vi "Pick&Place_ladder_shih_v5_peek.vi"() -> ()   [LabVIEW 2016]
uses:
  Classes/Controllers/I-O/Copy of NI-DAQ Folder/NI-DAQ.lvclass
  D:/INTT/V1/Classes/Controllers/I-O/Copy of I-O Folder/I-O.lvclass
  Classes/Controllers/Dispenser/Copy of Ultimus V2 Folder/Ultimus V2.lvclass
  <vilib>/Analysis/coordinate.llb/2D Cartesian Coordinate Rotation (Scalar).vi
  <vilib>/Utility/file.llb/Read Delimited Spreadsheet (DBL).vi
  <vilib>/Utility/file.llb/Write Delimited Spreadsheet (DBL).vi
  Classes/Controllers/Motion/Copy of Motion Folder/Motion.lvclass
  Classes/Controllers/Camera/Copy of Controller Folder/Controller.lvclass
  <vilib>/Analysis/NI_AALPro.lvlib
  Classes/Controllers/I-O/Copy of I-O Folder/I-O.lvclass
panel:
  out "chip distance":dbl format="%#_8g"
  out "after SL":dbl[](array[numeric]) format="%#_8g"
  in  "module placing offset":dbl[][](array[numeric])=[[0.0, -0.1, 0.0, 0.0], [0.0, -0.1, 0.0, 0.0]]
  out "after SR":dbl[](array[numeric]) format="%#_8g"
  out "after NL":dbl[](array[numeric]) format="%#_8g"
  out "S chip":dbl[](array[numeric]) format="%#_8g"
  out "N chip":dbl[](array[numeric]) format="%#_8g"
  in  "file path (dialog if empty) 2":path=path "C:/Users/PAGANIS/Desktop/shih cheng wei/OGP/test1-2.txt"
  out "bless from OGP !!! Center of  stave":dbl[](array[numeric])
  out "bless from OGP !! measured stave size":dbl[](array[numeric])
  in  "Bless from OGP":bool
  out "FROM Detail !!! Center of module on stave":dbl[](array[numeric])
  out "FROM Detail !! measured stave size":dbl[](array[numeric])
  in  "Align Stave in detail":bool
  in  "check height?":bool
  in  "Uttimus presssure":i64=10
  out "Status":bool
  out "measured HDI top-left position":dbl[][](array[numeric])
  in  "HDI vacuum channel":i32=18
  in  "vacuum":bool=TRUE
  in  "HDI vacuum":bool
  out "measured stave size":dbl[](array[numeric])
  out "Stave mark":dbl[][](array[numeric])
  out "Center of module on stave":dbl[](array[numeric])
  out "Center of HDI from alignment mark":dbl[](array[numeric])
  out "Measured HDI size":dbl[][](array[numeric])
  out "module position on stave":dbl[][](array[numeric])
  in  "Default Stave dimension":dbl[](array[numeric])=[34.0, 472.0, -0.335295, -0.000320234]
  in  "Default Stave upper left mark":dbl[](array[numeric])=[584.376, 675.576, 70.9882, 0.000840064]
  out "Needle parking position":dbl[](array[numeric])
  in  "Uppler / Lower Stave":bool=TRUE
  out "Gantry current position":dbl[](array[numeric])
  in  "READ Position":bool
  in  "Needle Height Compenstation\n(glue gap)":dbl=0.33
  in  "Needle Alignment":bool
  in  "Parking position":dbl[](array[numeric])=[625.0, 625.0, 0.0, 0.01]
  in  "GOTO":bool
  in  "Default Pickup Tool Position":dbl[][](array[numeric])=[[152.226, 682.729, 36.8129, -0.0151898], [700.0, 800.0, 20.0, 0.01]]
  in  "Number of module \nto be assembled":i32=1
  in  "Default HDI alignment \nmark position":dbl[](array[numeric])=[448.322, 976.582, 74.9872, 0.000191129]
  in  "Default HDI size":dbl[](array[numeric])=[24.2437, 231.446, -0.099339, 0.000191129]
  out "# of tasks excuted":i32
  out "module on tray position":dbl[][](array[numeric])
  out "PickupTool \nCenterPosition":dbl[](array[numeric])
  in  "Inititalize":bool
  in  "Pick and place":bool
  in  "Deposit Glue":bool
  in  "Measure Pickup Tools":bool
  in  "Align Stave":bool
  out "default module position on stave":dbl[][](array[numeric])
  in  "Stop":bool
  in  "Measure HDI":bool
  # "Ladder Assembly"
  # "Lower\nmodule"
  # "Upper\nmodule"
  # "Sensor 0.32 -> 200 micron glue thickness\nChips 0.37-> 140 micron glue thickness"
  # "ACTIONS"
  # "Stave infomation"
  # "Module infomation"
  # "Pick and Place"
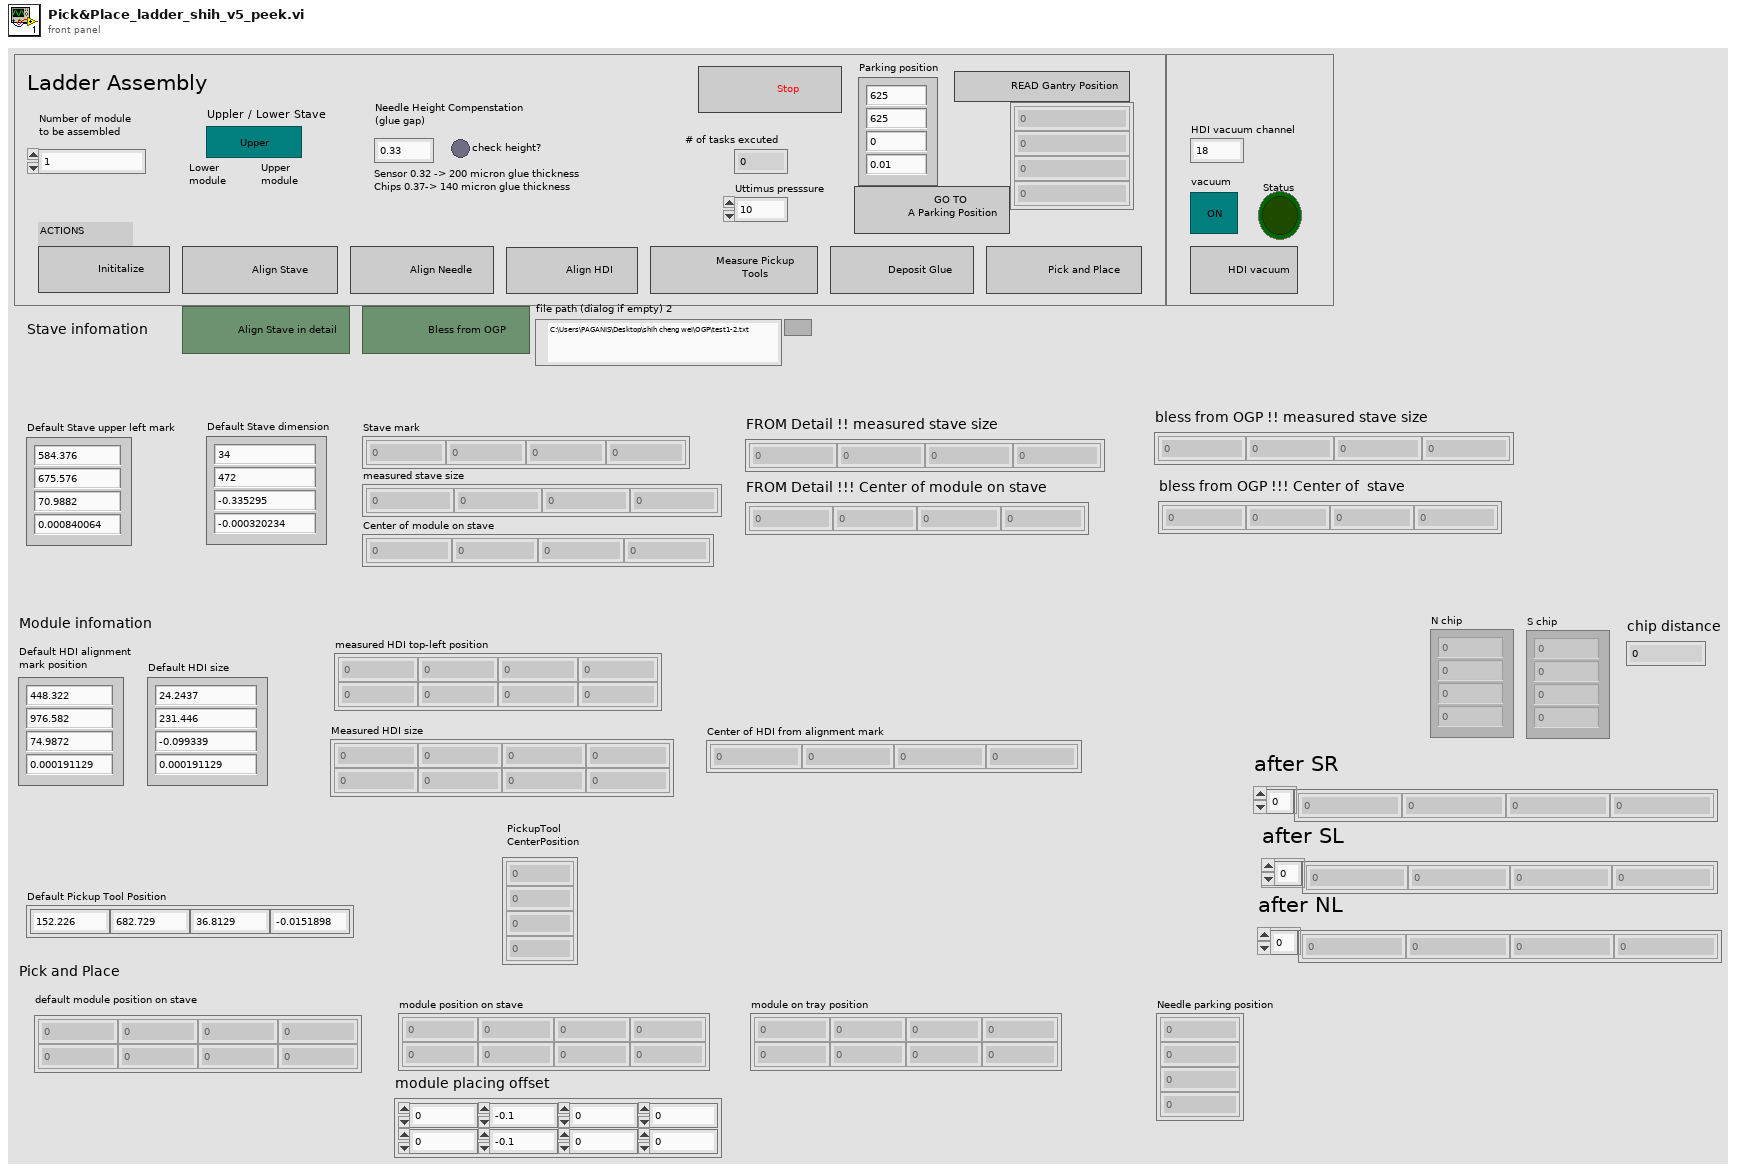
[diagram p1: front panel]
types:
  T1 = typedef "Controller.lvclass/Controllers.ctl" = cluster{"Copy of Motion.lvclass":refnum<class "Motion.lvclass">, "Copy of I-O.lvclass":refnum<class "I-O.lvclass">, "Copy of Dispenser.lvclass":refnum<class "Dispenser.lvclass">}
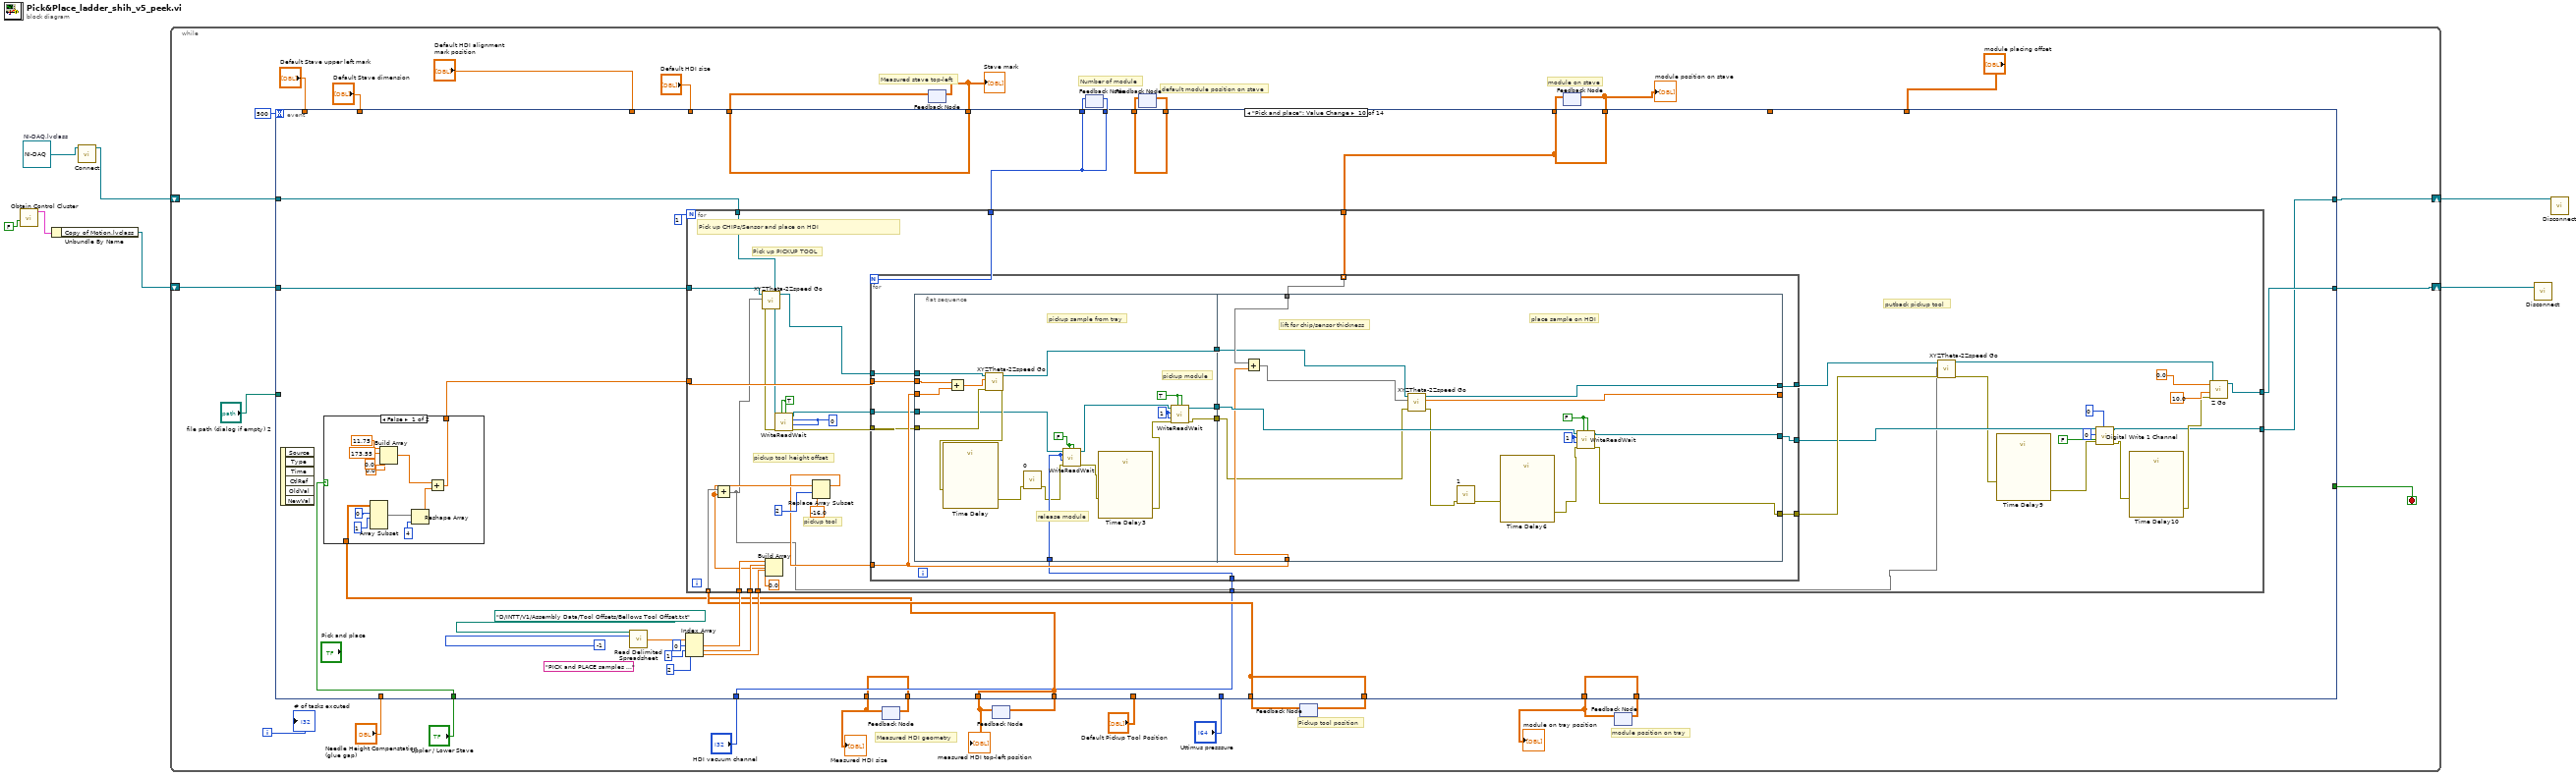
[diagram p0: block diagram]
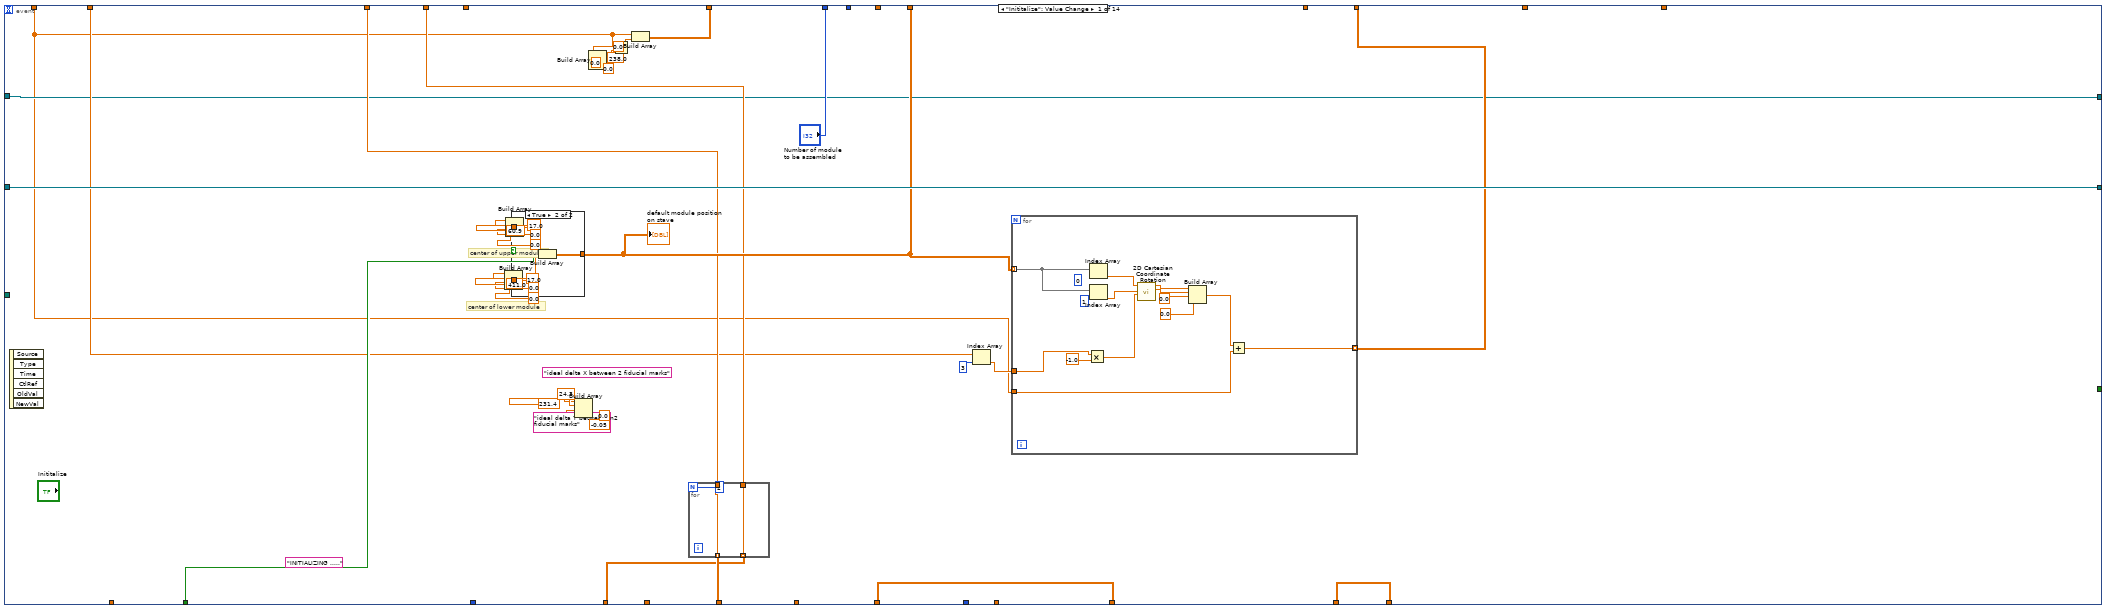
[diagram p2: hidden frame]
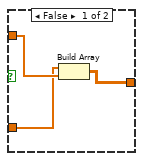
[diagram p3: hidden frame]
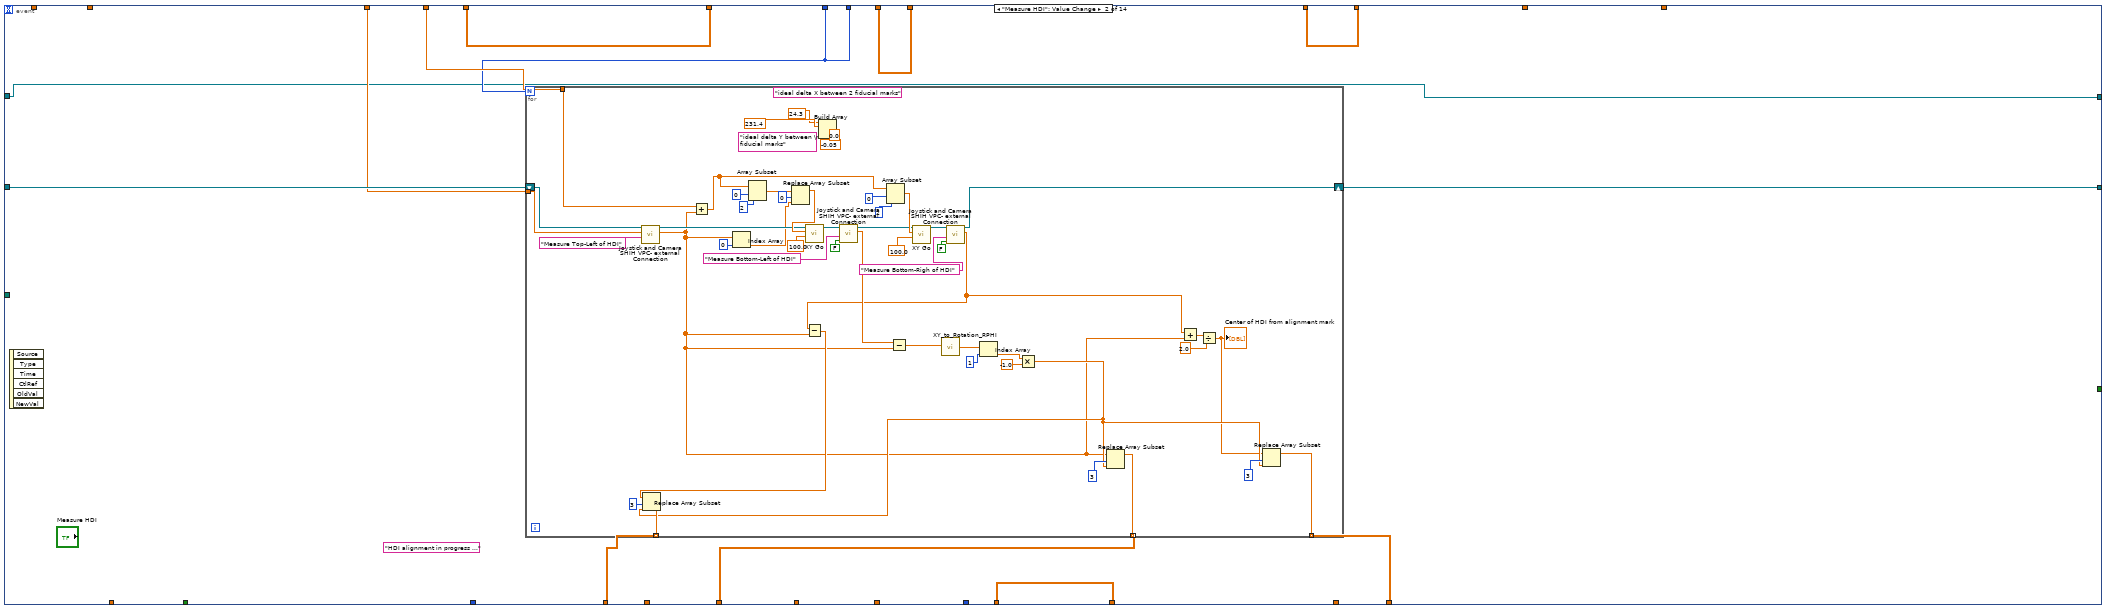
[diagram p4: hidden frame]
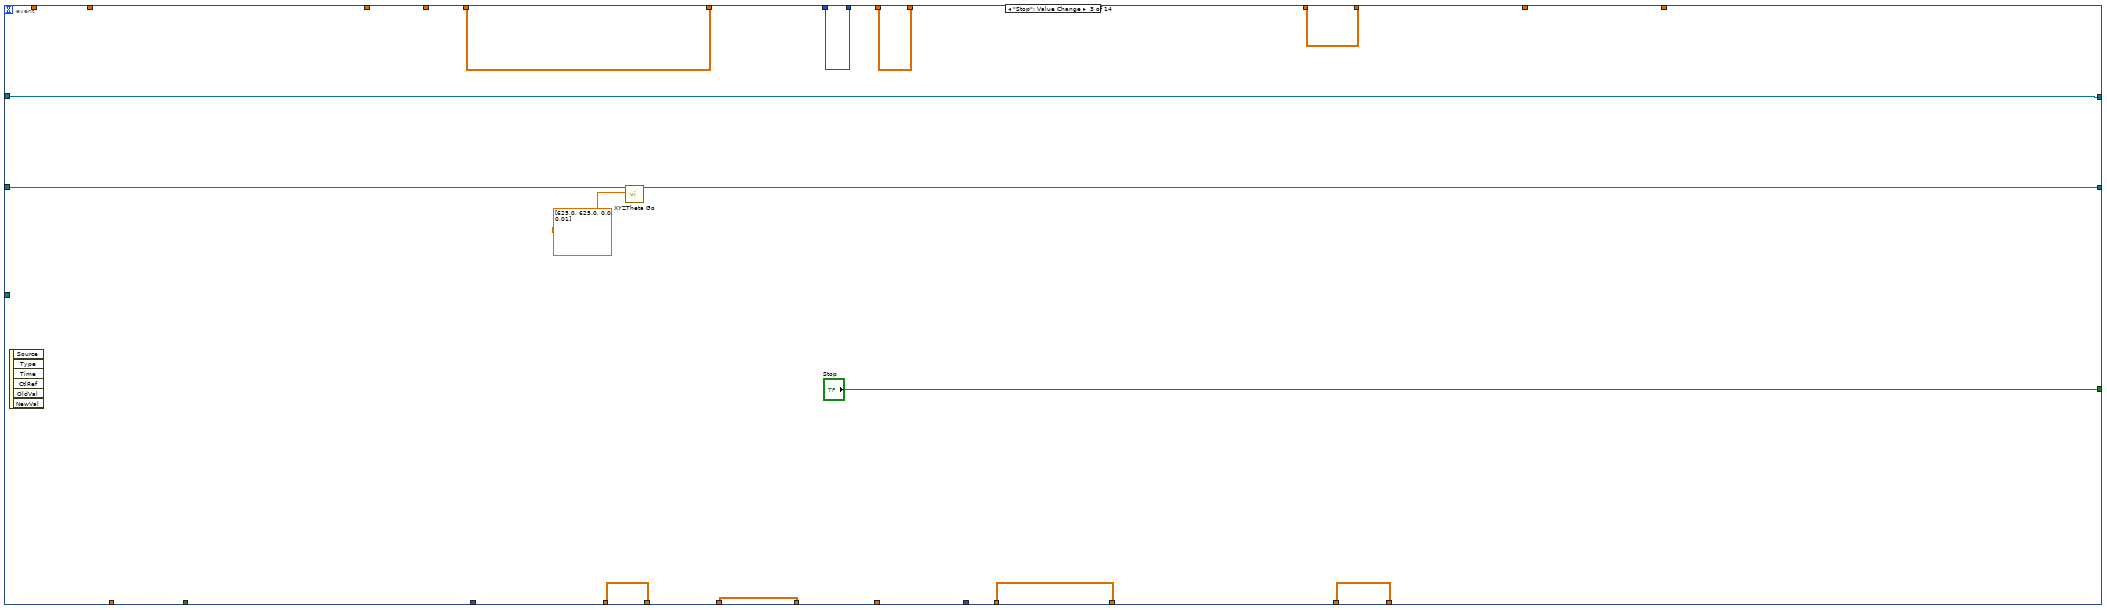
[diagram p5: hidden frame]
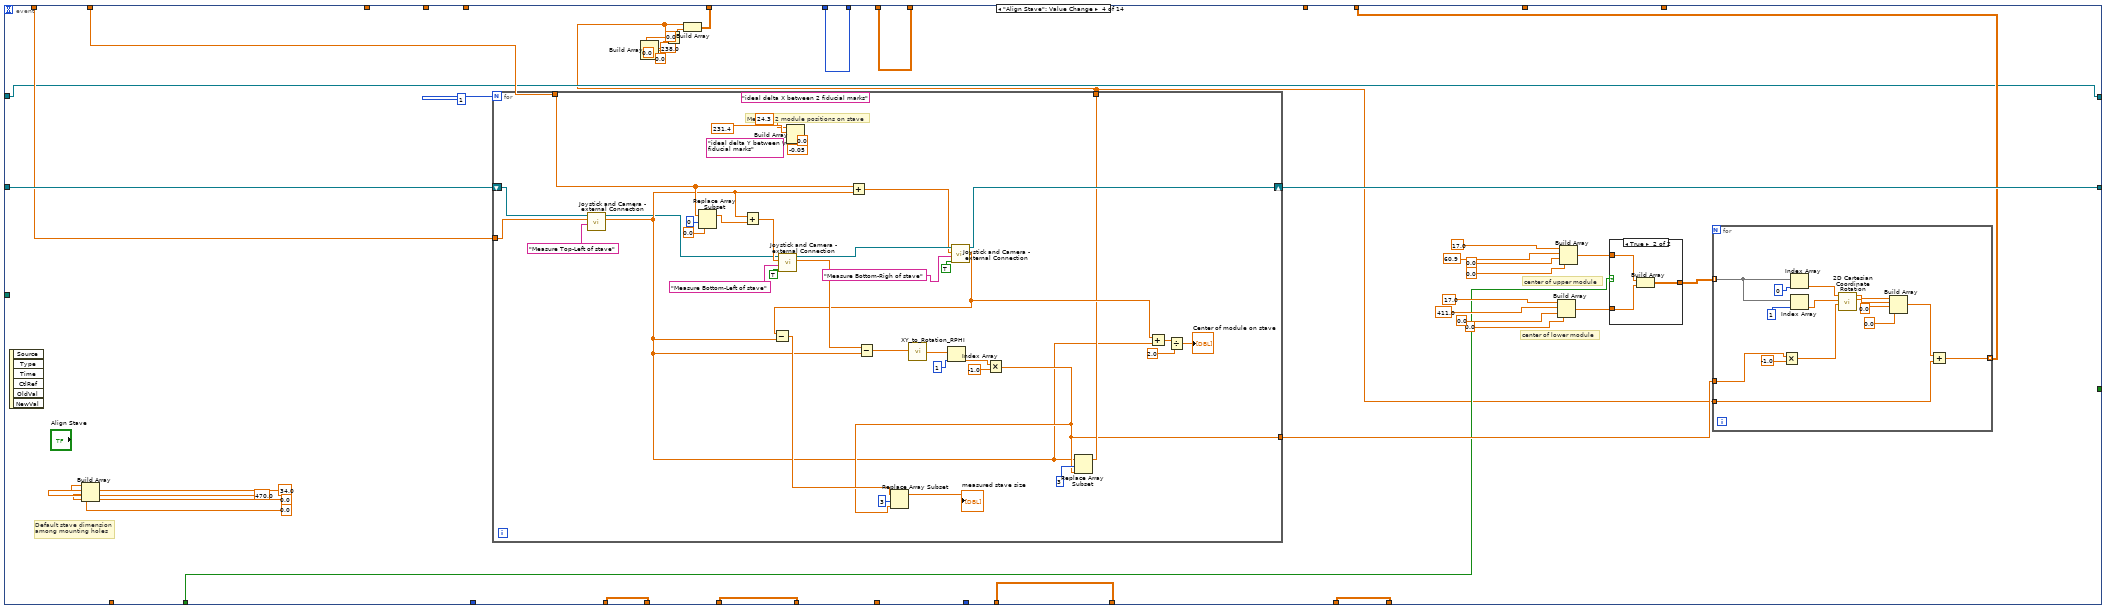
[diagram p6: hidden frame]
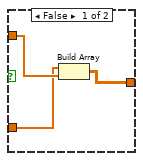
[diagram p7: hidden frame]
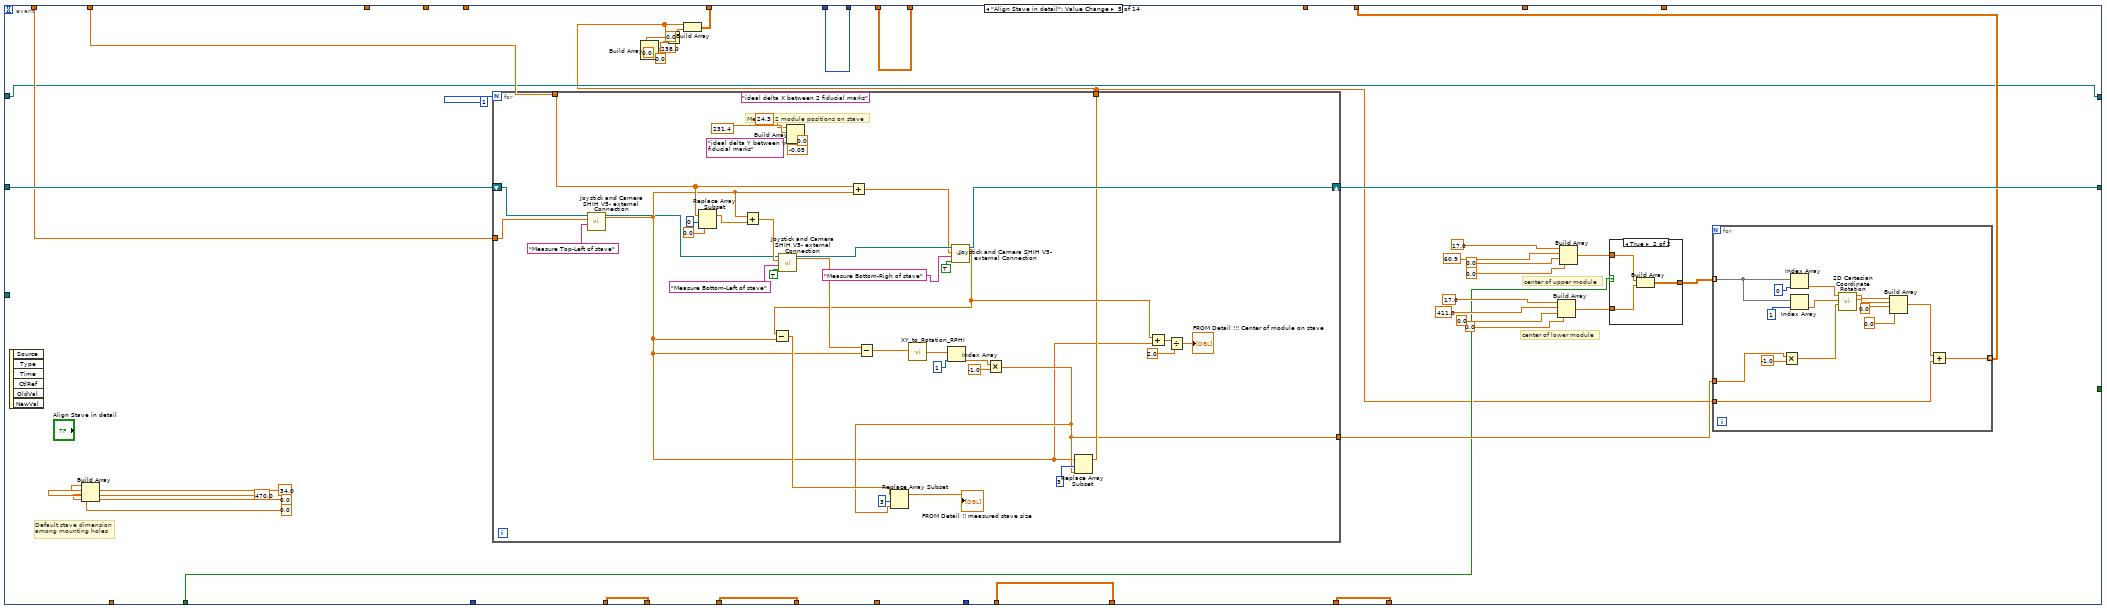
[diagram p8: hidden frame]
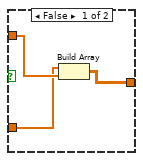
[diagram p9: hidden frame]
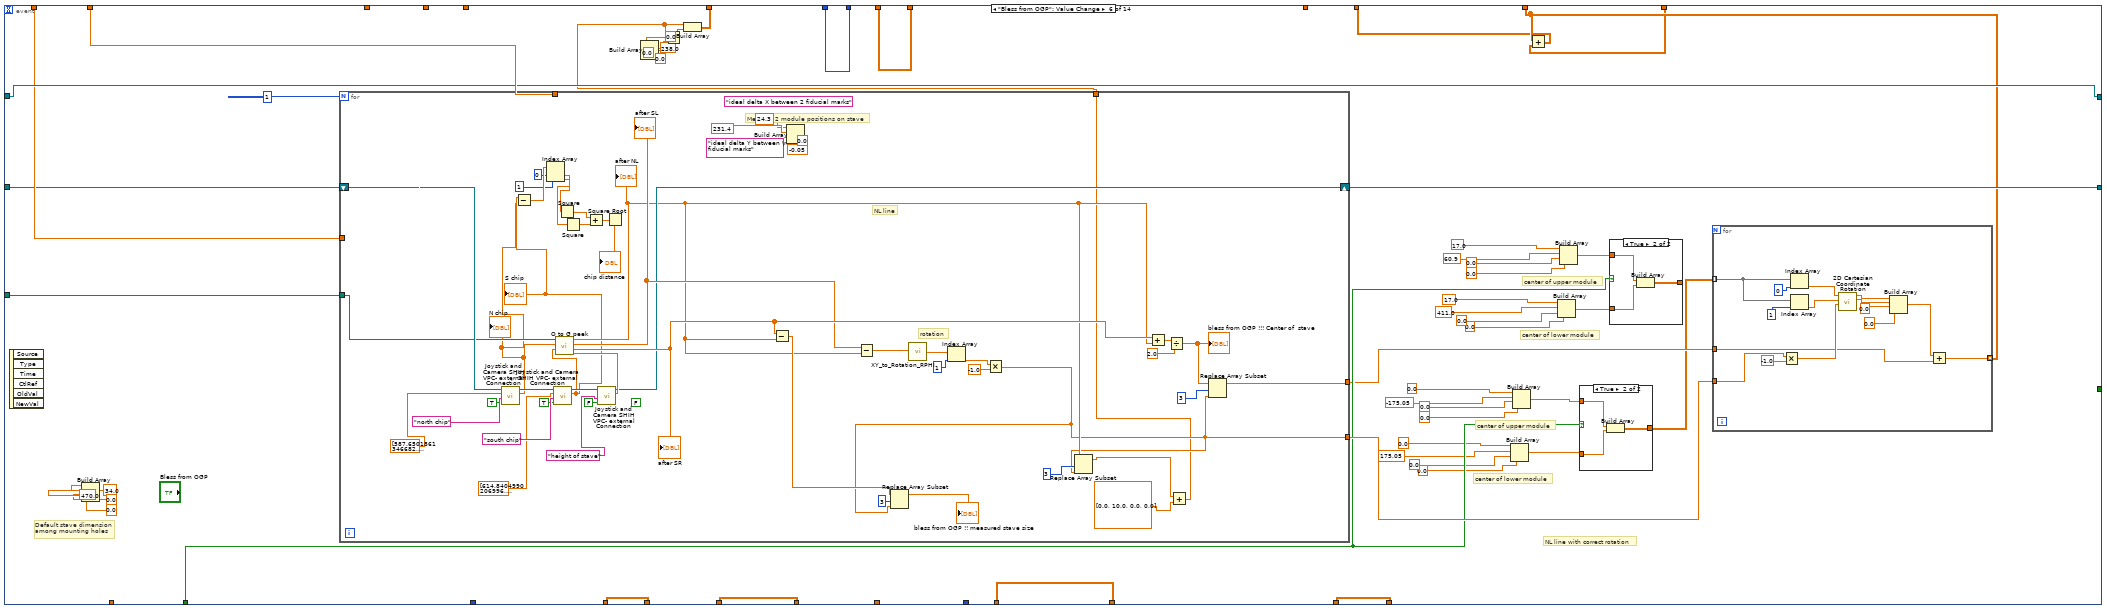
[diagram p10: hidden frame]
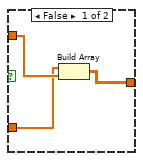
[diagram p11: hidden frame]
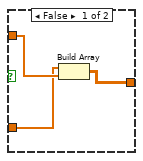
[diagram p12: hidden frame]
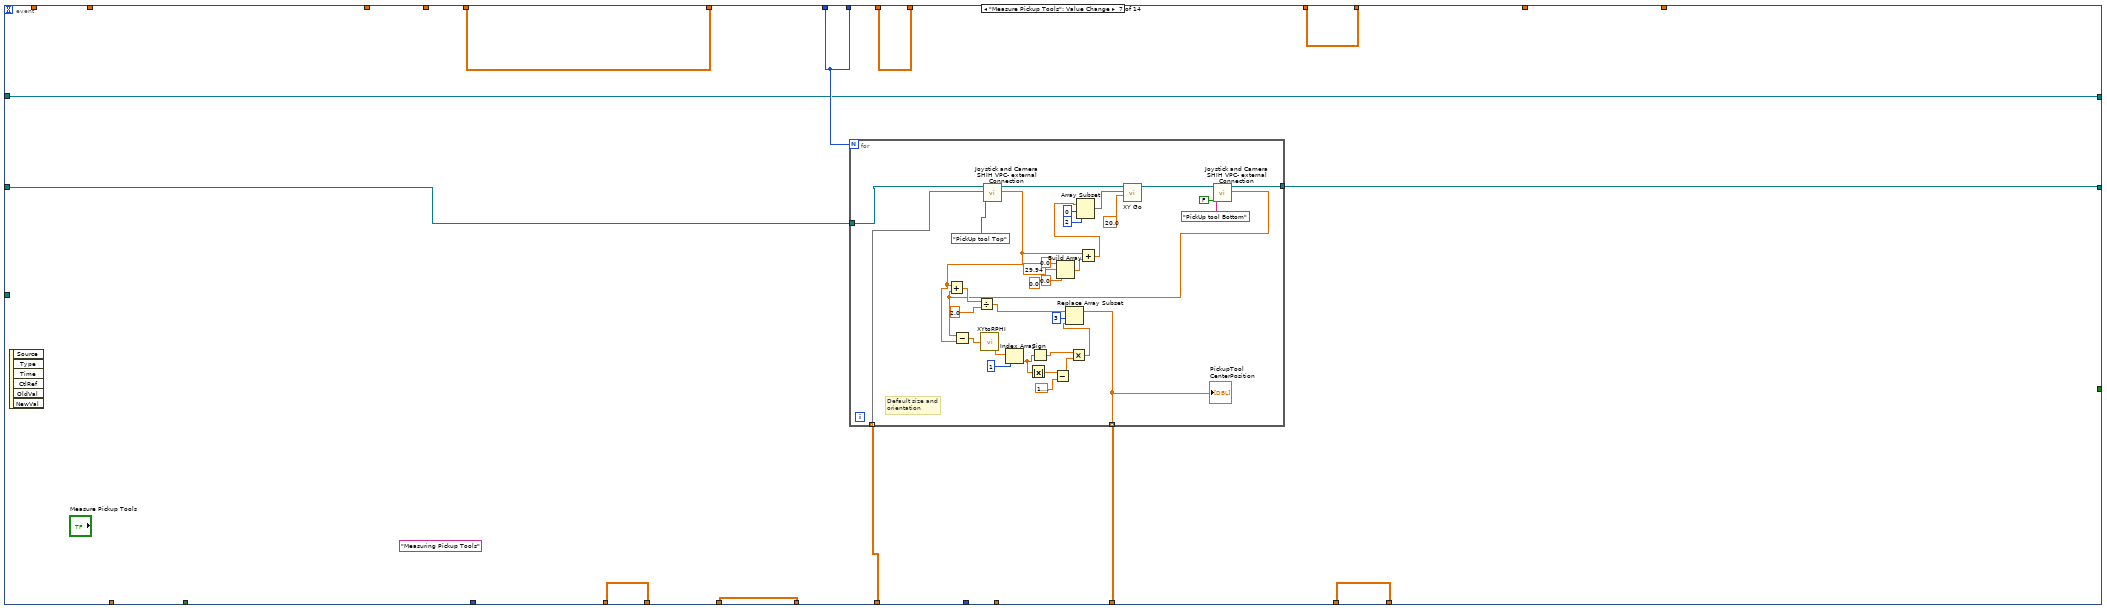
[diagram p13: hidden frame]
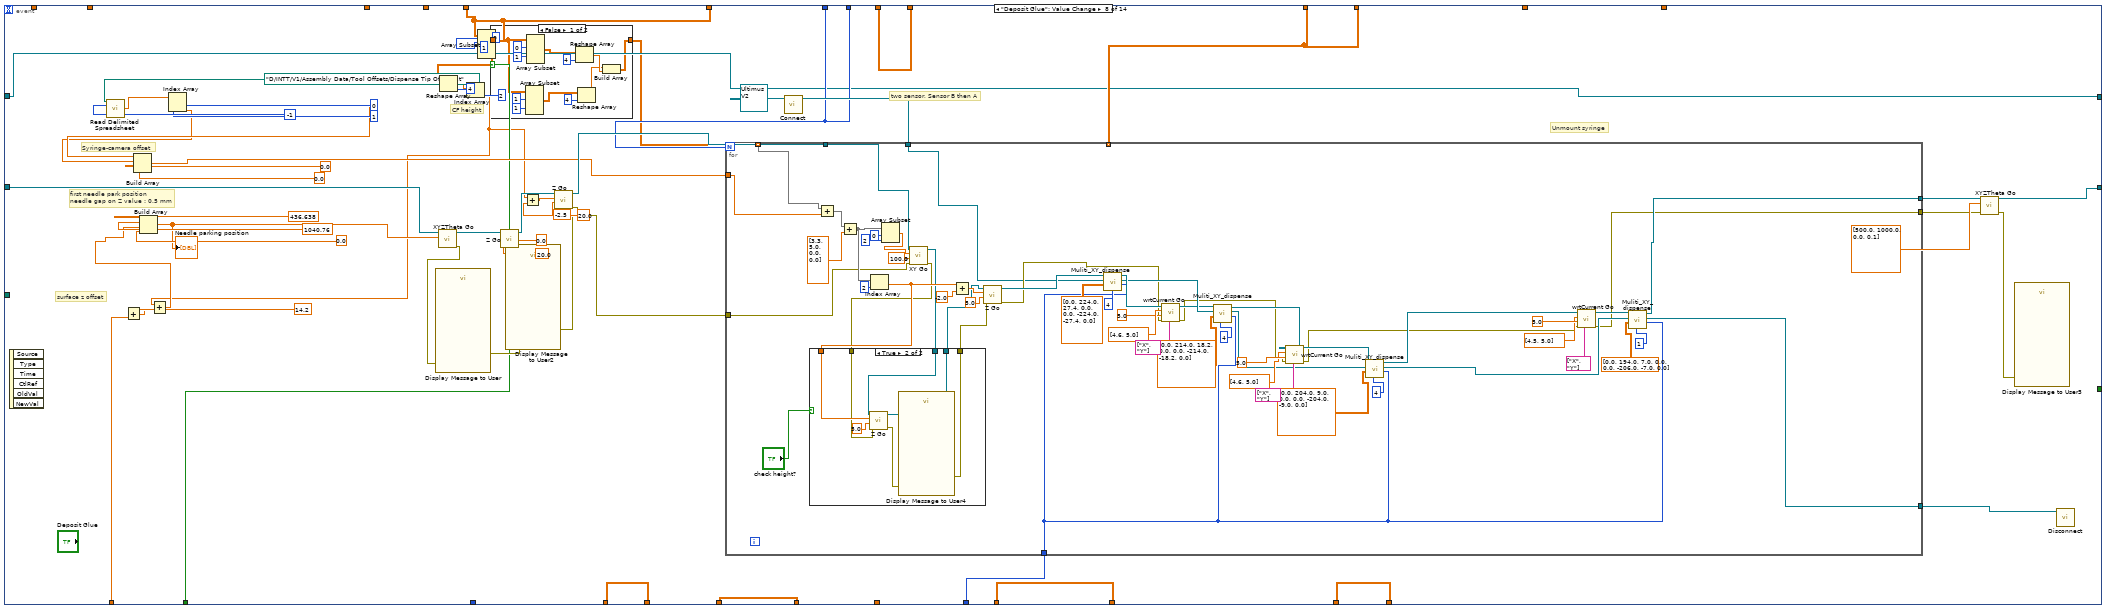
[diagram p14: hidden frame]
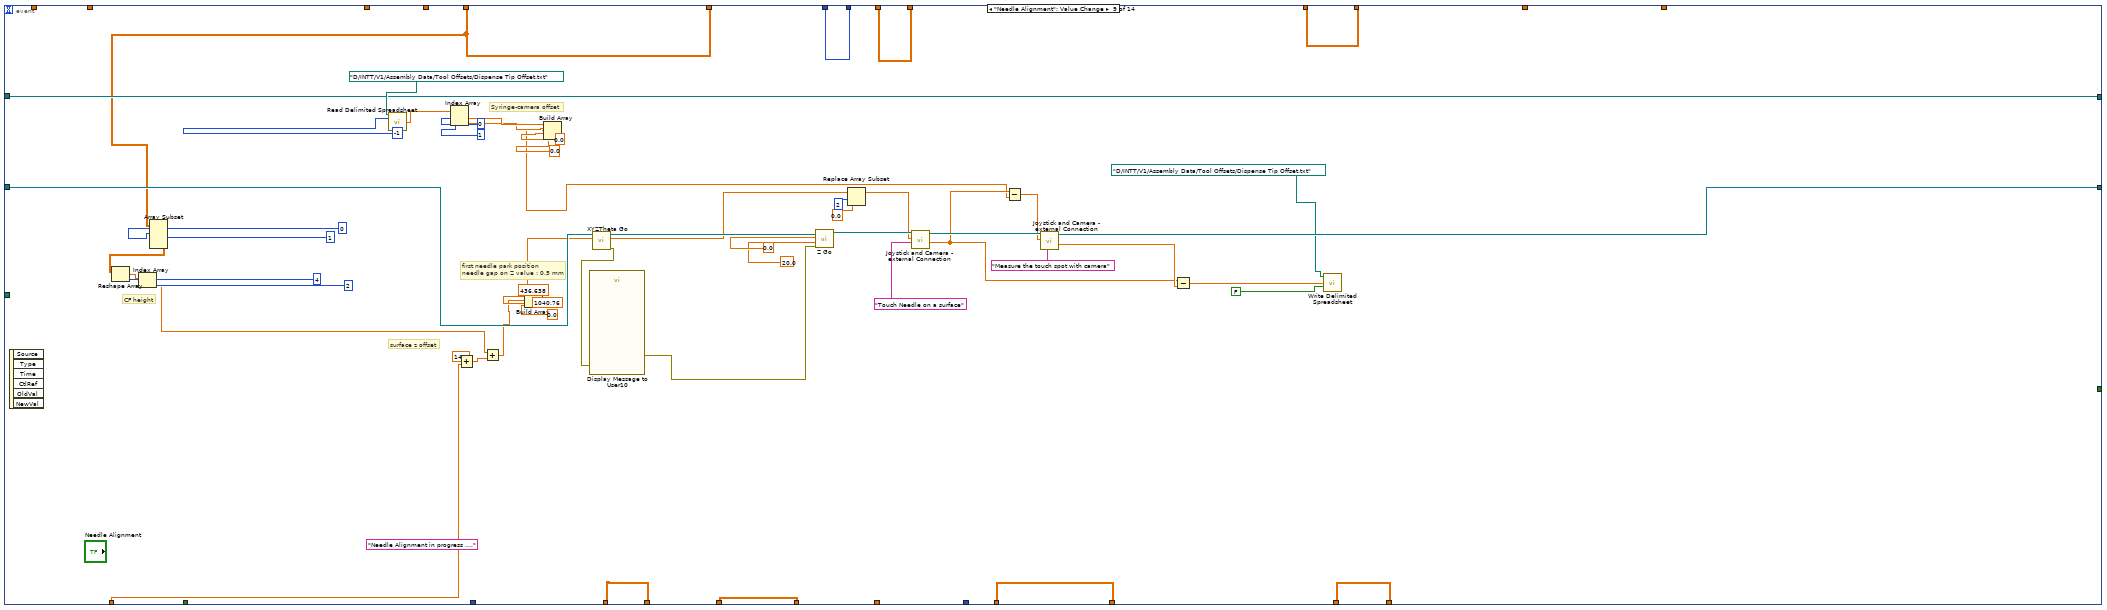
[diagram p17: hidden frame]
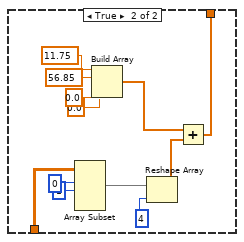
[diagram p18: hidden frame]
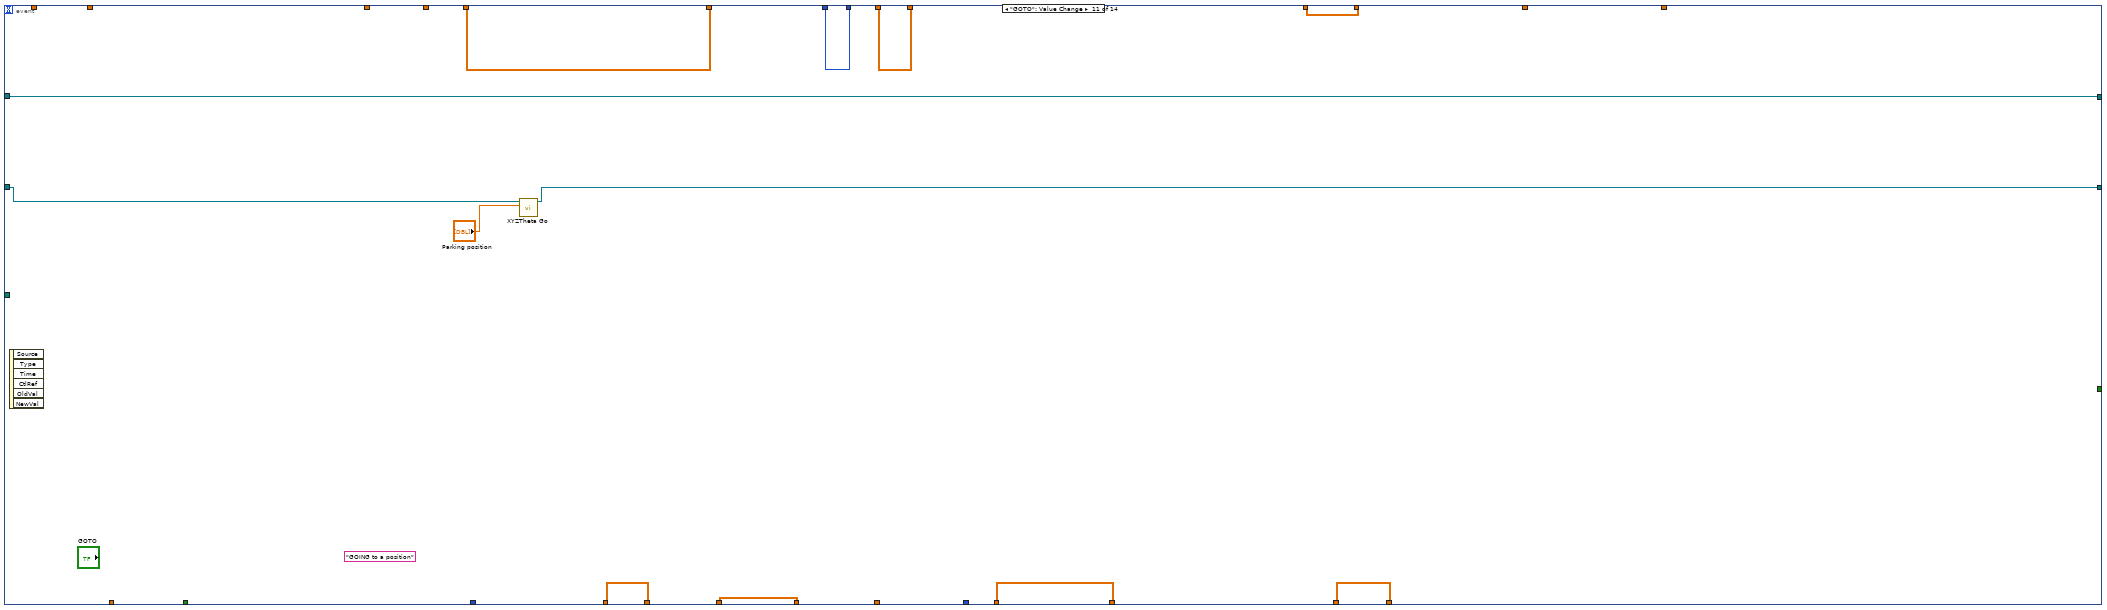
[diagram p19: hidden frame]
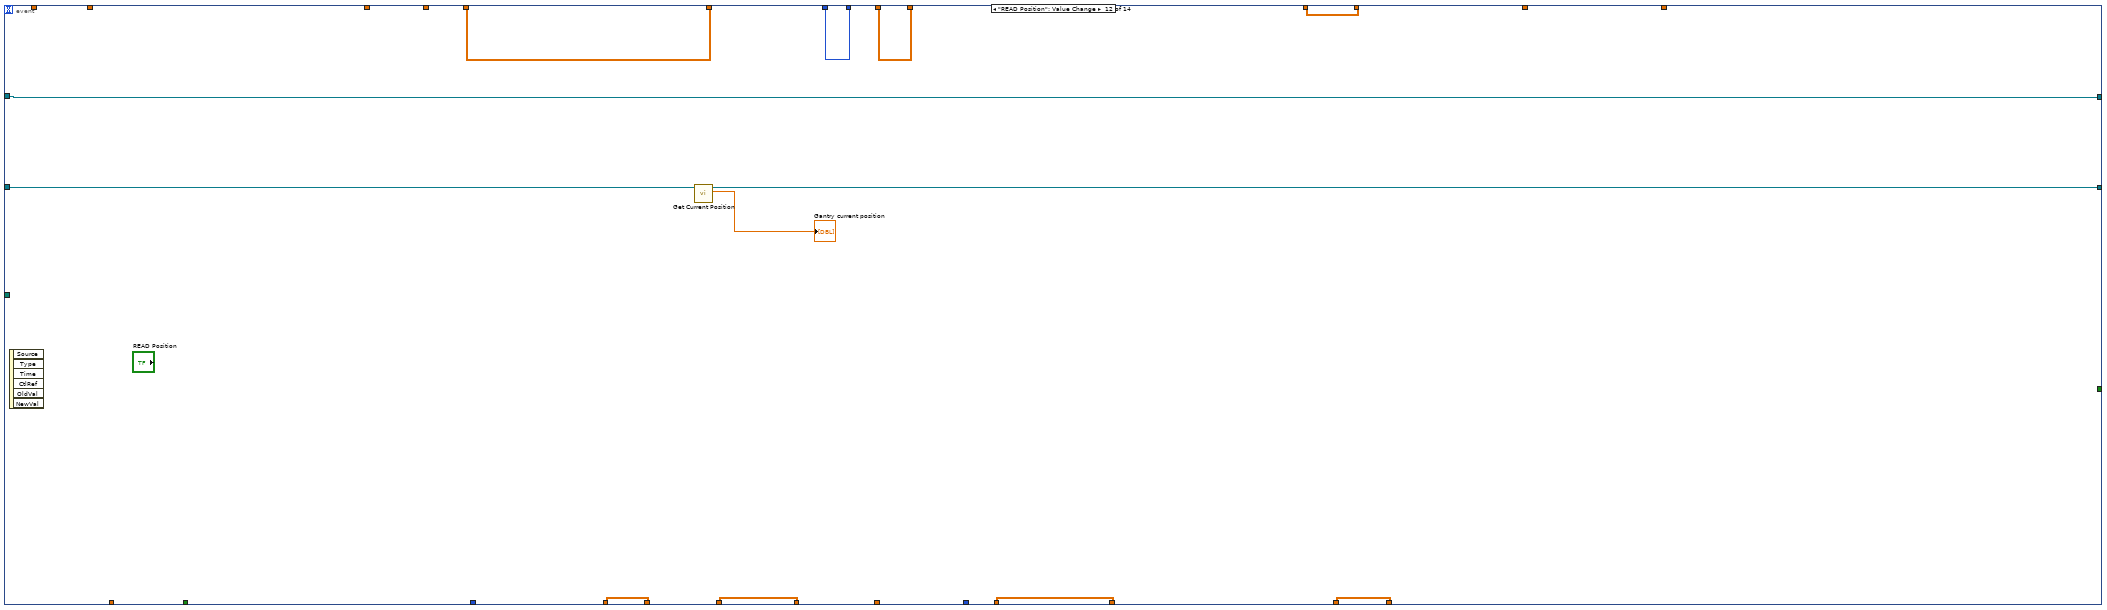
[diagram p20: hidden frame]
diagram:
  w3 = refnum<class "NI-DAQ.lvclass"> refnum  # NI-DAQ.lvclass
  n1 = call "Obtain Control Cluster.vi"("I/O"=FALSE) -> ("Control Out"=w7:T1)  [unwired: 10 in]
  n2 = Unbundle By Name(w7) -> ("Copy of Motion.lvclass"=w5:refnum<class "Motion.lvclass">)
  n3 = call-dynamic "Connect.vi"("NI-DAQ in"=w3) -> ("NI-DAQ out"=w2:refnum<class "NI-DAQ.lvclass">)  [unwired: 9 in, 1 out]
  n4 = while {
    shift-right: [w34] -> w4
    shift-left: w5 -> [w41]
    shift-right: [w13] -> w1
    shift-left: w2 -> [w17]
    i -> [w33]
    stop <- w40 stop-if-true
    # "default module position on stave"
    # "Pickup tool position"
    # "Number of module"
    # "Measured HDI geometry"
    # "module position on tray"
    # "Measured stave top-left"
    # "module on stave"
    n5 = feedback #1() -> (w38:dbl[][])  [unwired: 1 in]
    n6 = feedback #2() -> (w39:dbl[][])  [unwired: 1 in]
    n7 = feedback #3() -> (w14:dbl[][])  [unwired: 1 in]
    n8 = feedback #4() -> (w32:i32)  [unwired: 1 in]
    n9 = feedback #5() -> (w27:dbl[][])  [unwired: 1 in]
    n10 = feedback #6() -> (w35:dbl[][])  [unwired: 1 in]
    n11 = feedback #7() -> (w21:dbl[][])  [unwired: 1 in]
    n12 = feedback #8() -> (w25:dbl[][])  [unwired: 1 in]
    "module on tray position" <- w25
    n13 = event shown="[9] \"Pick and place\": Value Change" {
      selector: _ -> [_ _ _ _ _ _ _ _ _ _ _ _ _ _]
      dyn-events: _ -> [_ _ _ _ _ _ _ _ _ _ _ _ _ _]
      timeout: 500 -> [_ _ _ _ _ _ _ _ _ _ _ _ _ _]
      tunnel: w41 -> [w75 w114 w176 w206 w302 w385 w509 w582 w716 w760 w874 w892 w894 w915]
      tunnel: [_ _ "Stop" _ _ _ _ _ _ _ _ _ _ _] -> w40
      tunnel: [w42 w108 w171 w177 w273 w388 w504 w544 w682 w738 w880 w888 w902 w914] -> w18
      tunnel: w39 -> [_ w108 w171 _ _ _ w504 w544 w682 w738 w880 w888 w902 w914]
      tunnel: [w52 w106 w170 w202 w298 w410 w503 w568 w719 w741 w877 w887 w896 w912] -> w19
      tunnel: w38 -> [_ _ w170 w202 w298 w410 w503 w568 w719 w741 w877 w887 w896 w912]
      tunnel: w32 -> [_ w104 w173 w207 w303 w413 w500 w571 w721 w745 w879 w889 w900 w907]
      tunnel: [w57 w105 w168 w209 w305 w415 w502 w570 w717 w748 w875 w885 w898 w909] -> w37
      tunnel: w25 -> [w57 _ w168 w209 w305 w415 w502 w570 w717 w748 w875 w885 w898 w909]
      tunnel: [w73 w109 w169 w214 w310 w420 w508 w569 w718 w749 w876 w886 w897 w910] -> w36
      tunnel: w35 -> [_ w109 w169 w214 w310 w420 _ w569 w718 w749 w876 w886 w897 w910]
      tunnel: [w75 w113 w174 w203 w299 w411 w507 w572 w708 w750 w872 w891 w894 w915] -> w34
      tunnel: ["Number of module \nto be assembled" w104 w173 w207 w303 w413 w500 w571 w721 w745 w879 w889 w900 w907] -> w31
      tunnel: "Default HDI alignment \nmark position" -> [w55 w112 _ _ _ _ _ _ _ _ _ _ _ _]
      tunnel: "Default HDI size" -> [w54 w111 _ _ _ _ _ _ _ _ _ _ _ _]
      tunnel: [w62 w110 w172 w208 w304 w414 w505 w567 w720 w747 w878 w890 w901 w913] -> w28
      tunnel: w27 -> [_ w110 w172 w208 w304 w414 w505 w567 w720 w747 w878 w890 w901 w913]
      tunnel: "Default Pickup Tool Position" -> [w73 _ _ _ _ _ w506 _ _ _ _ _ _ _]
      tunnel: "Uppler / Lower Stave" -> [w58 _ _ w187 w283 w381 _ w552 _ w736 _ _ _ _]
      tunnel: "Default Stave upper left mark" -> [w43 _ _ w205 w301 w387 _ _ _ _ _ _ _ _]
      tunnel: "Default Stave dimension" -> [w51 _ _ w204 w300 w412 _ _ _ _ _ _ _ _]
      tunnel: [w59 w107 w166 w186 w282 w382 w501 w566 w699 w737 w870 w882 w899 w908] -> w20
      tunnel: w21 -> [_ w107 w166 _ _ _ w501 w566 w699 w737 w870 w882 w899 w908]
      tunnel: w17 -> [w50 w102 w164 w185 w281 w396 w498 w561 w697 w744 w869 w881 w906 w918]
      tunnel: [w50 w102 w164 w185 w281 w396 w498 w561 w697 w743 w869 w881 w893 w916] -> w13
      tunnel: "HDI vacuum channel" -> [_ _ _ _ _ _ _ _ _ w742 _ _ w903 w917]
      tunnel: [w53 w103 w165 w201 w297 w409 w499 w562 w698 w740 w871 w883 w895 w911] -> w15
      tunnel: w14 -> [_ _ w165 w201 w297 w409 w499 w562 w698 w740 w871 w883 w895 w911]
      tunnel: "Needle Height Compenstation\n(glue gap)" -> [_ _ _ _ _ _ _ w554 w690 _ _ _ _ _]
      tunnel: "Uttimus presssure" -> [_ _ _ _ _ _ _ w553 _ _ _ _ _ _]
      tunnel: "file path (dialog if empty) 2" -> [_ _ _ _ _ w386 _ _ _ _ _ _ _ _]
      tunnel: [_ _ _ _ _ w384 _ _ _ _ _ _ _ _] -> _
      tunnel: "module placing offset" -> [_ _ _ _ _ w383 _ _ _ _ _ _ _ _]
      event "Inititalize": Value Change {
        (unwired) "INITIALIZING ....." ("String")
        (unwired) "ideal delta Y between \n2 fiducial marks"
        (unwired) "ideal delta X between 2 fiducial marks"
        # "center of lower module"
        # "center of upper module"
        n14 = event-data() -> ()  [unwired: 1 in, 6 out]
        n15 = Build Array(17.0 ("element"), 411.0 ("element"), 0.0 ("element"), 0.0 ("element")) -> (w63:dbl[])
        n16 = Build Array(17.0 ("element"), 60.9 ("element"), 0.0 ("element"), 0.0 ("element")) -> (w64:dbl[])
        n17 = case shown="True" w58 {
          tunnel: w64 -> [w84 w87]
          tunnel: w63 -> [w83 w86]
          tunnel: [w82 w85] -> w62
          frame False {
            n18 = Build Array(w83, w84) -> (w82:dbl[][])
          }
          frame True {
            n19 = Build Array(w87, w86) -> (w85:dbl[][])
          }
        }
        "default module position on stave" <- w62
        n20 = Build Array(24.3 ("y"), 231.4 ("y"), 0.0 ("element"), -0.05 ("element")) -> ()  [unwired: 1 out]
        n21 = Build Array(0.0 ("element"), 238.0 ("element"), 0.0 ("element"), 0.0 ("element")) -> (w45:dbl[])
        n22 = Add(x=w43, y=w45) -> (x+y=w44:dbl[])
        n23 = Build Array(w43, w44) -> (w42:dbl[][])
        n24 = for {
          N: 2 -> [_]
          tunnel: w55 -> [w81]
          tunnel: [w81] -> w53 mode=indexing
          tunnel: w54 -> [w80]
          tunnel: [w80] -> w52 mode=indexing
        }
        n25 = Index Array(array=w51, index=3) -> (element=w60:dbl)
        n26 = for {
          tunnel: w62 -> [w95] mode=indexing
          tunnel: w60 -> [w89]
          tunnel: w43 -> [w94]
          tunnel: [w92] -> w59 mode=indexing
          (unwired) 0 ("index")
          n27 = Multiply(x=w89, y=-1.0) -> (x*y=w90:dbl)
          n28 = Index Array(array=w95) -> (element=w98:dbl)  [unwired: 1 in]
          n29 = Index Array(array=w95, index=1) -> (element=w97:dbl)
          n30 = call-poly <vilib>:"2D Cartesian Coordinate Rotation.vi"("theta"=w90, "y"=w97, "x"=w98) -> ("y out"=w100:dbl, "x out"=w99:dbl)  [unwired: 6 in, 1 out]
          n31 = Build Array(w99, w100, 0.0 ("element"), 0.0 ("element")) -> (w93:dbl[])
          n32 = Add(x=w93, y=w94) -> (x+y=w92:dbl[])
        }
      }
      event "Measure HDI": Value Change {
        (unwired) "HDI alignment in progress ..." ("String")
        n33 = event-data() -> ()  [unwired: 1 in, 6 out]
        n34 = for {
          N: w104 -> [_]
          tunnel: w111 -> [w126]
          shift-right: [w123] -> w113
          shift-left: w114 -> [w124]
          tunnel: w112 -> [w125]
          tunnel: [w160] -> w103 mode=indexing
          tunnel: [w159] -> w106 mode=indexing
          tunnel: [w116] -> w105 mode=indexing
          (unwired) "ideal delta Y between \n2 fiducial marks"
          (unwired) "ideal delta X between 2 fiducial marks"
          n35 = call "Joystick and Camera SHIH VPC- external Connection.vi"("Motion in"=w124, "XYZTheta"=w125, "Measurement Point"="Measure Top-Left of HDI") -> ("Motion out"=w139:refnum<class "Motion.lvclass">, "Sum"=w115:dbl[])  [unwired: 4 in, 2 out]
          n36 = Add(x=w126, y=w115) -> (x+y=w143:dbl[])
          n37 = Index Array(array=w115, index=0) -> (element=w130:dbl)
          n38 = Array Subset(array=w143, index=0, length=2) -> (w142:dbl[])
          n39 = Replace Array Subset(array=w142, new element=w130, index=0) -> (w140:dbl[])
          n40 = call-dynamic "XY Go.vi"("Speed"=100.0, "XY"=w140, "Motion in"=w139) -> ("Motion out"=w147:refnum<class "Motion.lvclass">)  [unwired: 7 in, 1 out]
          n41 = Build Array(24.3 ("y"), 231.4 ("y"), 0.0 ("element"), -0.05 ("element")) -> ()  [unwired: 1 out]
          n42 = call "Joystick and Camera SHIH VPC- external Connection.vi"("Motion in"=w147, "Measurement Point"="Measure Bottom-Left of HDI", "Inital GO"=FALSE) -> ("Motion out"=w138:refnum<class "Motion.lvclass">, "Sum"=w129:dbl[])  [unwired: 4 in, 2 out]
          n43 = Array Subset(array=w143, index=0, length=2) -> (w153:dbl[])
          n44 = Subtract(x=w129, y=w115) -> (x-y=w137:dbl[])
          n45 = call-dynamic "XY Go.vi"("Speed"=100.0, "XY"=w153, "Motion in"=w138) -> ("Motion out"=w157:refnum<class "Motion.lvclass">)  [unwired: 7 in, 1 out]
          n46 = call "XY_to_Rotation_RPHI.vi"("X-Y"=w137) -> ("r-phi"=w133:dbl[])
          n47 = call "Joystick and Camera SHIH VPC- external Connection.vi"("Motion in"=w157, "Measurement Point"="Measure Bottom-Righ of HDI", "Inital GO"=FALSE) -> ("Motion out"=w123:refnum<class "Motion.lvclass">, "Sum"=w120:dbl[])  [unwired: 4 in, 2 out]
          n48 = Subtract(x=w120, y=w115) -> (x-y=w121:dbl[])
          n49 = Index Array(array=w133, index=1) -> (element=w127:dbl)
          n50 = Multiply(x=w127, y=-1.0) -> (x*y=w118:dbl)
          n51 = Replace Array Subset(array=w121, new element=w118, index=3) -> (w159:dbl[])
          n52 = Replace Array Subset(array=w115, new element=w118, index=3) -> (w160:dbl[])
          n53 = Add(x=w120, y=w115) -> (x+y=w162:dbl[])
          n54 = Divide(x=w162, y=2.0) -> (x/y=w117:dbl[])
          "Center of HDI from alignment mark" <- w117
          n55 = Replace Array Subset(array=w117, new element=w118, index=3) -> (w116:dbl[])
        }
      }
      event "Stop": Value Change {
        n56 = event-data() -> ()  [unwired: 1 in, 6 out]
        n57 = call "XYZTheta Go.vi"("XYZTheta In"=dbl[] [625.0, 625.0, 0.0, 0.01], "Motion in"=w176) -> ("Motion out"=w174:refnum<class "Motion.lvclass">)  [unwired: 7 in, 2 out]
      }
      event "Align Stave": Value Change {
        # "center of lower module"
        # "center of upper module"
        # "Default stave dimension\namong mounting holes"
        # "Measure 2 module positions on stave"
        n58 = event-data() -> ()  [unwired: 1 in, 6 out]
        n59 = Build Array(34.0 ("element"), 470.0 ("element"), 0.0 ("element"), 0.0 ("element")) -> ()  [unwired: 1 out]
        n60 = for {
          N: 1 -> [_]
          tunnel: w204 -> [w221]
          shift-right: [w231] -> w203
          shift-left: w206 -> [w232]
          tunnel: w205 -> [w233]
          tunnel: [w226] -> w179
          tunnel: [w224] -> w189
          (unwired) "ideal delta Y between \n2 fiducial marks"
          (unwired) "ideal delta X between 2 fiducial marks"
          n61 = call "Joystick and Camera - external Connection.vi"("Motion in"=w232, "XYZTheta"=w233, "Measurement Point"="Measure Top-Left of stave") -> ("Motion out"=w215:refnum<class "Motion.lvclass">, "Sum"=w217:dbl[])  [unwired: 4 in, 2 out]
          n62 = Replace Array Subset(array=w221, new element=0.0 ("new element/subarray"), index=0) -> (w218:dbl[])
          n63 = Add(x=w217, y=w218) -> (x+y=w216:dbl[])
          n64 = call "Joystick and Camera - external Connection.vi"("Motion in"=w215, "XYZTheta"=w216, "Measurement Point"="Measure Bottom-Left of stave", "Inital GO"=TRUE) -> ("Motion out"=w223:refnum<class "Motion.lvclass">, "Sum"=w236:dbl[])  [unwired: 3 in, 2 out]
          n65 = Build Array(24.3 ("y"), 231.4 ("y"), 0.0 ("element"), -0.05 ("element")) -> ()  [unwired: 1 out]
          n66 = Add(x=w221, y=w217) -> (x+y=w222:dbl[])
          n67 = Subtract(x=w236, y=w217) -> (x-y=w242:dbl[])
          n68 = call "XY_to_Rotation_RPHI.vi"("X-Y"=w242) -> ("r-phi"=w238:dbl[])
          n69 = Index Array(array=w238, index=1) -> (element=w234:dbl)
          n70 = call "Joystick and Camera - external Connection.vi"("Motion in"=w223, "XYZTheta"=w222, "Measurement Point"="Measure Bottom-Righ of stave", "Inital GO"=TRUE) -> ("Motion out"=w231:refnum<class "Motion.lvclass">, "Sum"=w228:dbl[])  [unwired: 3 in, 2 out]
          n71 = Subtract(x=w228, y=w217) -> (x-y=w229:dbl[])
          n72 = Multiply(x=w234, y=-1.0) -> (x*y=w224:dbl)
          n73 = Replace Array Subset(array=w229, new element=w224, index=3) -> (→"measured stave size":dbl[])
          n74 = Replace Array Subset(array=w217, new element=w224, index=3) -> (w226:dbl[])
          n75 = Add(x=w228, y=w217) -> (x+y=w250:dbl[])
          n76 = Divide(x=w250, y=2.0) -> (x/y=→"Center of module on stave":dbl[])
        }
        n77 = Build Array(0.0 ("element"), 238.0 ("element"), 0.0 ("element"), 0.0 ("element")) -> (w180:dbl[])
        n78 = Add(x=w179, y=w180) -> (x+y=w178:dbl[])
        n79 = Build Array(w179, w178) -> (w177:dbl[][])
        n80 = Build Array(17.0 ("element"), 411.0 ("element"), 0.0 ("element"), 0.0 ("element")) -> (w191:dbl[])
        n81 = Build Array(17.0 ("element"), 60.9 ("element"), 0.0 ("element"), 0.0 ("element")) -> (w192:dbl[])
        n82 = case shown="True" w187 {
          tunnel: w192 -> [w269 w272]
          tunnel: w191 -> [w268 w271]
          tunnel: [w267 w270] -> w190
          frame False {
            n83 = Build Array(w268, w269) -> (w267:dbl[][])
          }
          frame True {
            n84 = Build Array(w272, w271) -> (w270:dbl[][])
          }
        }
        n85 = for {
          tunnel: w190 -> [w260] mode=indexing
          tunnel: w189 -> [w255]
          tunnel: w179 -> [w259]
          tunnel: [w257] -> w186 mode=indexing
          n86 = Multiply(x=w255, y=-1.0) -> (x*y=w254:dbl)
          n87 = Index Array(array=w260, index=0) -> (element=w263:dbl)
          n88 = Index Array(array=w260, index=1) -> (element=w262:dbl)
          n89 = call-poly <vilib>:"2D Cartesian Coordinate Rotation.vi"("theta"=w254, "y"=w262, "x"=w263) -> ("y out"=w265:dbl, "x out"=w264:dbl)  [unwired: 6 in, 1 out]
          n90 = Build Array(w264, w265, 0.0 ("element"), 0.0 ("element")) -> (w258:dbl[])
          n91 = Add(x=w258, y=w259) -> (x+y=w257:dbl[])
        }
      }
      event "Align Stave in detail": Value Change {
        # "center of lower module"
        # "center of upper module"
        # "Default stave dimension\namong mounting holes"
        # "Measure 2 module positions on stave"
        n92 = event-data() -> ()  [unwired: 1 in, 6 out]
        n93 = Build Array(34.0 ("element"), 470.0 ("element"), 0.0 ("element"), 0.0 ("element")) -> ()  [unwired: 1 out]
        n94 = for {
          N: 1 -> [_]
          tunnel: w300 -> [w317]
          shift-right: [w327] -> w299
          shift-left: w302 -> [w328]
          tunnel: w301 -> [w329]
          tunnel: [w322] -> w275
          tunnel: [w320] -> w285
          (unwired) "ideal delta Y between \n2 fiducial marks"
          (unwired) "ideal delta X between 2 fiducial marks"
          n95 = call "Joystick and Camera SHIH V5- external Connection.vi"("Motion in"=w328, "XYZTheta"=w329, "Measurement Point"="Measure Top-Left of stave") -> ("final out"=w313:dbl[], "Motion out"=w311:refnum<class "Motion.lvclass">)  [unwired: 5 in, 1 out]
          n96 = Replace Array Subset(array=w317, new element=0.0 ("new element/subarray"), index=0) -> (w314:dbl[])
          n97 = Add(x=w313, y=w314) -> (x+y=w312:dbl[])
          n98 = call "Joystick and Camera SHIH V5- external Connection.vi"("Motion in"=w311, "XYZTheta"=w312, "Measurement Point"="Measure Bottom-Left of stave", "Inital GO"=TRUE) -> ("final out"=w332:dbl[], "Motion out"=w319:refnum<class "Motion.lvclass">)  [unwired: 4 in, 1 out]
          n99 = Build Array(24.3 ("y"), 231.4 ("y"), 0.0 ("element"), -0.05 ("element")) -> ()  [unwired: 1 out]
          n100 = Add(x=w317, y=w313) -> (x+y=w318:dbl[])
          n101 = Subtract(x=w332, y=w313) -> (x-y=w338:dbl[])
          n102 = call "XY_to_Rotation_RPHI.vi"("X-Y"=w338) -> ("r-phi"=w334:dbl[])
          n103 = Index Array(array=w334, index=1) -> (element=w330:dbl)
          n104 = call "Joystick and Camera SHIH V5- external Connection.vi"("Motion in"=w319, "XYZTheta"=w318, "Measurement Point"="Measure Bottom-Righ of stave", "Inital GO"=TRUE) -> ("final out"=w324:dbl[], "Motion out"=w327:refnum<class "Motion.lvclass">)  [unwired: 4 in, 1 out]
          n105 = Subtract(x=w324, y=w313) -> (x-y=w325:dbl[])
          n106 = Multiply(x=w330, y=-1.0) -> (x*y=w320:dbl)
          n107 = Replace Array Subset(array=w325, new element=w320, index=3) -> (→"FROM Detail !! measured stave size":dbl[])
          n108 = Replace Array Subset(array=w313, new element=w320, index=3) -> (w322:dbl[])
          n109 = Add(x=w324, y=w313) -> (x+y=w346:dbl[])
          n110 = Divide(x=w346, y=2.0) -> (x/y=→"FROM Detail !!! Center of module on stave":dbl[])
        }
        n111 = Build Array(0.0 ("element"), 238.0 ("element"), 0.0 ("element"), 0.0 ("element")) -> (w276:dbl[])
        n112 = Add(x=w275, y=w276) -> (x+y=w274:dbl[])
        n113 = Build Array(w275, w274) -> (w273:dbl[][])
        n114 = Build Array(17.0 ("element"), 411.0 ("element"), 0.0 ("element"), 0.0 ("element")) -> (w287:dbl[])
        n115 = Build Array(17.0 ("element"), 60.9 ("element"), 0.0 ("element"), 0.0 ("element")) -> (w288:dbl[])
        n116 = case shown="True" w283 {
          tunnel: w288 -> [w365 w368]
          tunnel: w287 -> [w364 w367]
          tunnel: [w363 w366] -> w286
          frame False {
            n117 = Build Array(w364, w365) -> (w363:dbl[][])
          }
          frame True {
            n118 = Build Array(w368, w367) -> (w366:dbl[][])
          }
        }
        n119 = for {
          tunnel: w286 -> [w356] mode=indexing
          tunnel: w285 -> [w351]
          tunnel: w275 -> [w355]
          tunnel: [w353] -> w282 mode=indexing
          n120 = Multiply(x=w351, y=-1.0) -> (x*y=w350:dbl)
          n121 = Index Array(array=w356, index=0) -> (element=w359:dbl)
          n122 = Index Array(array=w356, index=1) -> (element=w358:dbl)
          n123 = call-poly <vilib>:"2D Cartesian Coordinate Rotation.vi"("theta"=w350, "y"=w358, "x"=w359) -> ("y out"=w361:dbl, "x out"=w360:dbl)  [unwired: 6 in, 1 out]
          n124 = Build Array(w360, w361, 0.0 ("element"), 0.0 ("element")) -> (w354:dbl[])
          n125 = Add(x=w354, y=w355) -> (x+y=w353:dbl[])
        }
      }
      event "Bless from OGP": Value Change {
        # "center of lower module"
        # "center of upper module"
        # "NL line with correct rotation"
        # "center of lower module"
        # "center of upper module"
        # "Default stave dimension\namong mounting holes"
        # "Measure 2 module positions on stave"
        n126 = event-data() -> ()  [unwired: 1 in, 6 out]
        n127 = Build Array(34.0 ("element"), 470.0 ("element"), 0.0 ("element"), 0.0 ("element")) -> ()  [unwired: 1 out]
        n128 = for {
          N: 1 -> [_]
          tunnel: w412 -> [_]
          shift-right: [w448] -> w411
          shift-left: w385 -> [w461]
          tunnel: w387 -> [_]
          tunnel: [w438] -> w390
          tunnel: [w442] -> w398
          tunnel: w386 -> [w450]
          tunnel: [w441] -> w370
          (unwired) FALSE ("Inital GO")
          (unwired) "ideal delta Y between \n2 fiducial marks"
          (unwired) "ideal delta X between 2 fiducial marks"
          # "NL line"
          # "rotation"
          n129 = call "Joystick and Camera SHIH VPC- external Connection.vi"("Motion in"=w461, "XYZTheta"=dbl[] [587.6501861346682, 659.8354057217969, 70.1155335060548, 0.010000094994154989] ("N chip"), "Measurement Point"="north chip", "Inital GO"=TRUE) -> ("Motion out"=w458:refnum<class "Motion.lvclass">, "Sum"=w436:dbl[])  [unwired: 3 in, 2 out]
          "N chip" <- w436
          n130 = call "Joystick and Camera SHIH VPC- external Connection.vi"("Motion in"=w458, "XYZTheta"=dbl[] [614.8404990206996, 1158.7590823829282, 70.34521582498871, 0.010000670236950445] ("S chip"), "Measurement Point"="south chip", "Inital GO"=TRUE) -> ("Motion out"=w457:refnum<class "Motion.lvclass">, "Sum"=w437:dbl[])  [unwired: 3 in, 2 out]
          "S chip" <- w437
          n131 = Subtract(x=w437, y=w436) -> (x-y=w435:dbl[])
          n132 = Index Array(array=w435, index #1=0 ("index"), index #2=1 ("index")) -> (element #1=w432:dbl, element #2=w431:dbl)
          n133 = Square(x=w432) -> (x^2=w429:dbl)
          n134 = Square(x=w431) -> (x^2=w430:dbl)
          n135 = Add(x=w429, y=w430) -> (x+y=w428:dbl)
          n136 = call "Joystick and Camera SHIH VPC- external Connection.vi"("Motion in"=w457, "Measurement Point"="height of stave", "Inital GO"=FALSE) -> ("Motion out"=w448:refnum<class "Motion.lvclass">, "Sum"=w449:dbl[])  [unwired: 4 in, 2 out]
          n137 = call "O to G peek.vi"("height"=w449, "south chip"=w437, "north chip"=w436, "Input file"=w450) -> ("output BR"=w452:dbl[], "output BL"=w451:dbl[], "output TL"=w445:dbl[])  [unwired: 4 in, 1 out]
          "after NL" <- w445
          "after SR" <- w452
          "after SL" <- w451
          n138 = Square Root(x=w428) -> (sqrt(x)=→"chip distance":dbl)
          n139 = Subtract(x=w452, y=w445) -> (x-y=w463:dbl[])
          n140 = Build Array(24.3 ("y"), 231.4 ("y"), 0.0 ("element"), -0.05 ("element")) -> ()  [unwired: 1 out]
          n141 = Subtract(x=w451, y=w445) -> (x-y=w469:dbl[])
          n142 = call "XY_to_Rotation_RPHI.vi"("X-Y"=w469) -> ("r-phi"=w468:dbl[])
          n143 = Index Array(array=w468, index=1) -> (element=w465:dbl)
          n144 = Multiply(x=w465, y=-1.0) -> (x*y=w442:dbl)
          n145 = Replace Array Subset(array=w463, new element=w442, index=3) -> (→"bless from OGP !! measured stave size":dbl[])
          n146 = Replace Array Subset(array=w445, new element=w442, index=3) -> (w439:dbl[])
          n147 = Add(x=w452, y=w445) -> (x+y=w475:dbl[])
          n148 = Divide(x=w475, y=2.0) -> (x/y=w443:dbl[])
          "bless from OGP !!! Center of  stave" <- w443
          n149 = Add(x=w439, y=dbl[] [0.0, 10.0, 0.0, 0.0]) -> (x+y=w438:dbl[])
          n150 = Replace Array Subset(array=w443, new element=w442, index=3) -> (w441:dbl[])
        }
        n151 = Build Array(0.0 ("element"), 238.0 ("element"), 0.0 ("element"), 0.0 ("element")) -> (w391:dbl[])
        n152 = Add(x=w390, y=w391) -> (x+y=w389:dbl[])
        n153 = Build Array(w390, w389) -> (w388:dbl[][])
        n154 = Build Array(0.0 ("element"), 175.05 ("element"), 0.0 ("element"), 0.0 ("element")) -> (w371:dbl[])
        n155 = Build Array(0.0 ("element"), -175.05 ("element"), 0.0 ("element"), 0.0 ("element")) -> (w372:dbl[])
        n156 = Build Array(17.0 ("element"), 411.0 ("element"), 0.0 ("element"), 0.0 ("element")) -> (w399:dbl[])
        n157 = Build Array(17.0 ("element"), 60.9 ("element"), 0.0 ("element"), 0.0 ("element")) -> (w400:dbl[])
        n158 = case shown="True" w381 {
          tunnel: w372 -> [w423 w426]
          tunnel: w371 -> [w422 w425]
          tunnel: [w421 w424] -> w369
          frame False {
            n159 = Build Array(w422, w423) -> (w421:dbl[][])
          }
          frame True {
            n160 = Build Array(w426, w425) -> (w424:dbl[][])
          }
        }
        n161 = case shown="True" w381 {
          tunnel: w400 -> [w494 w497]
          tunnel: w399 -> [w493 w496]
          tunnel: [w492 w495] -> _
          frame False {
            n162 = Build Array(w493, w494) -> (w492:dbl[][])
          }
          frame True {
            n163 = Build Array(w497, w496) -> (w495:dbl[][])
          }
        }
        n164 = for {
          tunnel: w369 -> [w485] mode=indexing
          tunnel: w398 -> [w481]
          tunnel: [w483] -> w384 mode=indexing
          tunnel: w370 -> [w477]
          n165 = Multiply(x=w481, y=-1.0) -> (x*y=w480:dbl)
          n166 = Index Array(array=w485, index=0) -> (element=w488:dbl)
          n167 = Index Array(array=w485, index=1) -> (element=w487:dbl)
          n168 = call-poly <vilib>:"2D Cartesian Coordinate Rotation.vi"("theta"=w480, "y"=w487, "x"=w488) -> ("y out"=w490:dbl, "x out"=w489:dbl)  [unwired: 6 in, 1 out]
          n169 = Build Array(w489, w490, 0.0 ("element"), 0.0 ("element")) -> (w484:dbl[])
          n170 = Add(x=w484, y=w477) -> (x+y=w483:dbl[])
        }
        n171 = Add(x=w384, y=w383) -> (x+y=w382:dbl[][])
      }
      event "Measure Pickup Tools": Value Change {
        (unwired) "Measuring Pickup Tools" ("String")
        n172 = event-data() -> ()  [unwired: 1 in, 6 out]
        n173 = for {
          N: w500 -> [_]
          tunnel: [w533] -> w508 mode=indexing
          tunnel: w509 -> [w537]
          tunnel: [w519] -> w507
          tunnel: w506 -> [w518] mode=indexing
          # "Default size and\norientation"
          n174 = call "Joystick and Camera SHIH VPC- external Connection.vi"("Motion in"=w537, "XYZTheta"=w518, "Measurement Point"="PickUp tool Top") -> ("Motion out"=w513:refnum<class "Motion.lvclass">, "Sum"=w536:dbl[])  [unwired: 4 in, 2 out]
          n175 = Build Array(0.0 ("element"), 29.94 ("element"), 0.0 ("element"), 0.0 ("element")) -> (w524:dbl[])
          n176 = Add(x=w536, y=w524) -> (x+y=w510:dbl[])
          n177 = Array Subset(array=w510, index=0, length=2) -> (w511:dbl[])
          n178 = call-dynamic "XY Go.vi"("Speed"=20.0, "XY"=w511, "Motion in"=w513) -> ("Motion out"=w512:refnum<class "Motion.lvclass">)  [unwired: 7 in, 1 out]
          n179 = call "Joystick and Camera SHIH VPC- external Connection.vi"("Motion in"=w512, "Measurement Point"="PickUp tool Bottom", "Inital GO"=FALSE) -> ("Motion out"=w519:refnum<class "Motion.lvclass">, "Sum"=w535:dbl[])  [unwired: 4 in, 2 out]
          n180 = Add(x=w536, y=w535) -> (x+y=w542:dbl[])
          n181 = Subtract(x=w535, y=w536) -> (x-y=w534:dbl[])
          n182 = Divide(x=w542, y=2.0) -> (x/y=w539:dbl[])
          n183 = call "XYtoRPHI.vi"("X-Y"=w534) -> ("r-phi"=w540:dbl[])
          n184 = Index Array(array=w540, index=1) -> (element=w528:dbl)
          n185 = Absolute Value(x=w528) -> (abs(x)=w531:dbl)
          n186 = Sign(1:w528) -> (0:w529:dbl)
          n187 = Subtract(x=w531, y=1.5707963267948966) -> (x-y=w530:dbl)
          n188 = Multiply(x=w529, y=w530) -> (x*y=w527:dbl)
          n189 = Replace Array Subset(array=w539, new element=w527, index=3) -> (w533:dbl[])
          "PickupTool \nCenterPosition" <- w533
        }
      }
      event "Deposit Glue": Value Change {
        # "CF height"
        # "surface z offset"
        # "two sensor, Sensor B then A"
        # "Unmount syringe"
        # "first needle park position\nneedle gap on Z value : 0.5 mm"
        # "Syringe-camera offset"
        n190 = event-data() -> ()  [unwired: 1 in, 6 out]
        n191 = call-poly <vilib>:"Read Delimited Spreadsheet.vi"("file path (dialog if empty)"=path "D:/INTT/V1/Assembly Data/Tool Offsets/Dispense Tip Offset.txt", "number of rows (all:-1)"=-1) -> ("first row"=w598:dbl[])  [unwired: 8 in, 5 out]
        n192 = Add(x=14.2 ("element"), y=w554) -> (x+y=w548:dbl)
        n193 = Index Array(array=w598, index #1=0 ("index"), index #2=1 ("index")) -> (element #1=w593:dbl, element #2=w591:dbl)
        n194 = Build Array(w593, w591, 0.0 ("element"), 0.0 ("element")) -> (w577:dbl[])
        n195 = Array Subset(array=w544, index (row)=0, length (row)=1 ("length")) -> (w557:dbl[][])  [unwired: 2 in]
        n196 = Reshape Array(w557, 4 ("dimension size")) -> (w550:dbl[])
        n197 = Index Array(array=w550, index=2) -> (element=w545:dbl)
        n198 = Add(x=w545, y=w548) -> (x+y=w547:dbl)
        n199 = Build Array(436.638, 1040.76, w547, 0.0 ("element")) -> (w546:dbl[])
        "Needle parking position" <- w546
        n200 = call "XYZTheta Go.vi"("XYZTheta In"=w546, "Motion in"=w582) -> ("error out"=w590:errorcluster, "Motion out"=w581:refnum<class "Motion.lvclass">)  [unwired: 7 in, 1 out]
        n201 = call "Display Message to User"("error in (no error)"=w590) -> ("error out"=w583:errorcluster)  [unwired: 9 in, 1 out]
        n202 = case shown="False" w552 {
          tunnel: w544 -> [w606 w615]
          tunnel: [w603 w615] -> w551
          frame False {
            n203 = Array Subset(array=w606, index (row)=1 ("index"), length (row)=1 ("length")) -> (w607:dbl[][])  [unwired: 2 in]
            n204 = Array Subset(array=w606, index (row)=0 ("index"), length (row)=1 ("length")) -> (w610:dbl[][])  [unwired: 2 in]
            n205 = Reshape Array(w610, 4 ("dimension size")) -> (w605:dbl[])
            n206 = Reshape Array(w607, 4 ("dimension size")) -> (w604:dbl[])
            n207 = Build Array(w604, w605) -> (w603:dbl[][])
          }
          frame True {
          }
        }
        n208 = call-dynamic "Z Go.vi"("error in (no error)"=w583, "Speed"=20.0, "Position"=0.0, "Motion in"=w581) -> ("error out"=w580:errorcluster, "Motion out"=w586:refnum<class "Motion.lvclass">)  [unwired: 6 in]
        n209 = call "Display Message to User2"("error in (no error)"=w580) -> ("error out"=w579:errorcluster)  [unwired: 9 in, 1 out]
        n210 = Add(x=w545, y=-2.5) -> (x+y=w587:dbl)
        n211 = call-dynamic "Z Go.vi"("error in (no error)"=w579, "Speed"=20.0, "Position"=w587, "Motion in"=w586) -> ("error out"=w556:errorcluster, "Motion out"=w578:refnum<class "Motion.lvclass">)  [unwired: 6 in]
        n212 = call-dynamic "Connect.vi"("Ultimus V in"=refnum<class "Ultimus V2.lvclass"> refnum ("Ultimus V2.lvclass")) -> ("Ultimus V out"=w576:refnum<class "Ultimus V2.lvclass">)  [unwired: 9 in, 1 out]
        n213 = for {
          N: w571 -> [_]
          tunnel: w578 -> [w630]
          tunnel: w576 -> [w629]
          tunnel: w577 -> [w631]
          tunnel: w566 -> [_] mode=indexing
          tunnel: w551 -> [w632] mode=indexing
          tunnel: [w628] -> w564
          tunnel: [w627] -> w563
          tunnel: w556 -> [w623]
          tunnel: [w624] -> w555
          tunnel: w553 -> [w622]
          (unwired) 100.0 ("Speed")
          n214 = Add(x=w632, y=w631) -> (x+y=w662:dbl[])
          n215 = Add(x=w662, y=dbl[] [3.3, 5.0, 0.0, 0.0]) -> (x+y=w663:dbl[])
          n216 = Index Array(array=w663, index=2) -> (element=w620:dbl)
          n217 = Array Subset(array=w663, index=0, length=2) -> (w638:dbl[])
          n218 = call-dynamic "XY Go.vi"("error in (no error)"=w623, "Speed"=100.0, "XY"=w638, "Motion in"=w630) -> ("error out"=w618:errorcluster, "Motion out"=w619:refnum<class "Motion.lvclass">)  [unwired: 6 in]
          n219 = case shown="True" "check height?" {
            tunnel: w620 -> [_ w679]
            tunnel: w619 -> [w672 w678]
            tunnel: w618 -> [w673 w677]
            tunnel: [w673 w675] -> w617
            tunnel: [w672 w674] -> w616
            frame False {
            }
            frame True {
              n220 = call-dynamic "Z Go.vi"("error in (no error)"=w677, "Speed"=5.0, "Position"=w679, "Motion in"=w678) -> ("error out"=w676:errorcluster, "Motion out"=w674:refnum<class "Motion.lvclass">)  [unwired: 6 in]
              n221 = call "Display Message to User4"("error in (no error)"=w676) -> ("error out"=w675:errorcluster)  [unwired: 9 in, 1 out]
            }
          }
          n222 = Add(x=w620, y=-2.0) -> (x+y=w637:dbl)
          n223 = call-dynamic "Z Go.vi"("error in (no error)"=w617, "Speed"=5.0, "Position"=w637, "Motion in"=w616) -> ("error out"=w635:errorcluster, "Motion out"=w636:refnum<class "Motion.lvclass">)  [unwired: 6 in]
          n224 = call "Muliti_XY_dispense.vi"("Pressure"=w622, "Path count"=4, "distances"=dbl[][] [[0.0, 224.0], [27.4, 0.0], [0.0, -224.0], [-27.4, 0.0]], "Ultimus V in"=w629, "Motion in"=w636) -> ("Ultimus V out"=w656:refnum<class "Ultimus V2.lvclass">, "Motion out"=w661:refnum<class "Motion.lvclass">)  [unwired: 5 in]
          n225 = call-dynamic "wrtCurrent Go.vi"("axis names"=string[] ["X", "Y"], "error in (no error)"=w635, "Speed"=5.0, "distances"=dbl[] [4.6, 5.0], "Motion in"=w661) -> ("error out"=w626:errorcluster, "Motion out"=w655:refnum<class "Motion.lvclass">)  [unwired: 5 in]
          n226 = call "Muliti_XY_dispense.vi"("Pressure"=w622, "Path count"=4, "distances"=dbl[][] [[0.0, 214.0], [18.2, 0.0], [0.0, -214.0], [-18.2, 0.0]], "Ultimus V in"=w656, "Motion in"=w655) -> ("Ultimus V out"=w648:refnum<class "Ultimus V2.lvclass">, "Motion out"=w647:refnum<class "Motion.lvclass">)  [unwired: 5 in]
          n227 = call-dynamic "wrtCurrent Go.vi"("axis names"=string[] ["X", "Y"], "error in (no error)"=w626, "Speed"=5.0, "distances"=dbl[] [4.6, 5.0], "Motion in"=w647) -> ("error out"=w625:errorcluster, "Motion out"=w646:refnum<class "Motion.lvclass">)  [unwired: 5 in]
          n228 = call "Muliti_XY_dispense.vi"("Pressure"=w622, "Path count"=4, "distances"=dbl[][] [[0.0, 204.0], [9.0, 0.0], [0.0, -204.0], [-9.0, 0.0]], "Ultimus V in"=w648, "Motion in"=w646) -> ("Ultimus V out"=w633:refnum<class "Ultimus V2.lvclass">, "Motion out"=w634:refnum<class "Motion.lvclass">)  [unwired: 5 in]
          n229 = call-dynamic "wrtCurrent Go.vi"("axis names"=string[] ["X", "Y"], "error in (no error)"=w625, "Speed"=5.0, "distances"=dbl[] [4.5, 5.0], "Motion in"=w634) -> ("error out"=w624:errorcluster, "Motion out"=w640:refnum<class "Motion.lvclass">)  [unwired: 5 in]
          n230 = call "Muliti_XY_dispense.vi"("Pressure"=w622, "Path count"=1, "distances"=dbl[][] [[0.0, 194.0], [7.0, 0.0], [0.0, -206.0], [-7.0, 0.0]], "Ultimus V in"=w633, "Motion in"=w640) -> ("Ultimus V out"=w627:refnum<class "Ultimus V2.lvclass">, "Motion out"=w628:refnum<class "Motion.lvclass">)  [unwired: 5 in]
        }
        n231 = call "XYZTheta Go.vi"("error in (no error)"=w555, "XYZTheta In"=dbl[] [500.0, 1000.0, 0.0, 0.1], "Motion in"=w564) -> ("error out"=w574:errorcluster, "Motion out"=w572:refnum<class "Motion.lvclass">)  [unwired: 6 in, 1 out]
        n232 = call "Display Message to User3"("error in (no error)"=w574) -> ()  [unwired: 9 in, 2 out]
        n233 = call-dynamic "Disconnect.vi"("Ultimus V in"=w563) -> ()  [unwired: 9 in, 1 out]
      }
      event "Needle Alignment": Value Change {
        (unwired) "Needle Alignment in progress ...." ("String")
        # "CF height"
        # "surface z offset"
        # "first needle park position\nneedle gap on Z value : 0.5 mm"
        # "Syringe-camera offset"
        n234 = event-data() -> ()  [unwired: 1 in, 6 out]
        n235 = Array Subset(array=w682, index (row)=0, length (row)=1 ("length")) -> (w685:dbl[][])  [unwired: 2 in]
        n236 = Reshape Array(w685, 4 ("dimension size")) -> (w684:dbl[])
        n237 = Index Array(array=w684, index=2) -> (element=w681:dbl)
        n238 = call-poly <vilib>:"Read Delimited Spreadsheet.vi"("file path (dialog if empty)"=path "D:/INTT/V1/Assembly Data/Tool Offsets/Dispense Tip Offset.txt", "number of rows (all:-1)"=-1) -> ("first row"=w732:dbl[])  [unwired: 8 in, 5 out]
        n239 = Index Array(array=w732, index #1=0 ("index"), index #2=1 ("index")) -> (element #1=w727:dbl, element #2=w726:dbl)
        n240 = Add(x=14.2 ("element"), y=w690) -> (x+y=w692:dbl)
        n241 = Add(x=w681, y=w692) -> (x+y=w691:dbl)
        n242 = Build Array(436.638, 1040.76, w691, 0.0 ("element")) -> (w689:dbl[])
        n243 = Build Array(w727, w726, 0.0 ("element"), 0.0 ("element")) -> (w701:dbl[])
        n244 = call "XYZTheta Go.vi"("XYZTheta In"=w689, "Motion in"=w716) -> ("error out"=w725:errorcluster, "XYZTheta Out"=w706:dbl[], "Motion out"=w715:refnum<class "Motion.lvclass">)  [unwired: 7 in]
        n245 = call "Display Message to User10"("error in (no error)"=w725) -> ("error out"=w722:errorcluster)  [unwired: 9 in, 1 out]
        n246 = call-dynamic "Z Go.vi"("error in (no error)"=w722, "Speed"=20.0, "Position"=0.0, "Motion in"=w715) -> ("Motion out"=w714:refnum<class "Motion.lvclass">)  [unwired: 6 in, 1 out]
        n247 = Replace Array Subset(array=w706, new element=0.0 ("new element/subarray"), index=2) -> (w703:dbl[])
        n248 = call "Joystick and Camera - external Connection.vi"("Motion in"=w714, "XYZTheta"=w703, "Measurement Point"="Touch Needle on a surface") -> ("Motion out"=w712:refnum<class "Motion.lvclass">, "Gantry"=w702:dbl[])  [unwired: 4 in, 2 out]
        n249 = Subtract(x=w702, y=w701) -> (x-y=w700:dbl[])
        n250 = call "Joystick and Camera - external Connection.vi"("Motion in"=w712, "XYZTheta"=w700, "Measurement Point"="Measure the touch spot with camera") -> ("Motion out"=w708:refnum<class "Motion.lvclass">, "Gantry"=w711:dbl[])  [unwired: 4 in, 2 out]
        n251 = Subtract(x=w702, y=w711) -> (x-y=w710:dbl[])
        n252 = call-poly <vilib>:"Write Delimited Spreadsheet.vi"("file path (dialog if empty)"=path "D:/INTT/V1/Assembly Data/Tool Offsets/Dispense Tip Offset.txt", "1D data"=w710, "append to file? (new file:F)"=FALSE) -> ()  [unwired: 11 in, 2 out]
      }
      event "Pick and place": Value Change {
        (unwired) "PICK and PLACE samples ..." ("String")
        n253 = event-data() -> ()  [unwired: 1 in, 6 out]
        n254 = case shown="False" w736 {
          tunnel: w740 -> [w846 w868]
          tunnel: [w845 w867] -> w739
          frame False {
            n255 = Array Subset(array=w846, index (row)=0 ("index"), length (row)=1 ("length")) -> (w848:dbl[][])  [unwired: 2 in]
            n256 = Build Array(11.75 ("element"), 173.55 ("element"), 0.0 ("element"), 0.0 ("element")) -> (w852:dbl[])
            n257 = Reshape Array(w848, 4 ("dimension size")) -> (w847:dbl[])
            n258 = Add(x=w852, y=w847) -> (x+y=w845:dbl[])
          }
          frame True {
            n259 = Array Subset(array=w868, index (row)=0 ("index"), length (row)=1 ("length")) -> (w858:dbl[][])  [unwired: 2 in]
            n260 = Build Array(11.75 ("element"), 56.85 ("element"), 0.0 ("element"), 0.0 ("element")) -> (w862:dbl[])
            n261 = Reshape Array(w858, 4 ("dimension size")) -> (w857:dbl[])
            n262 = Add(x=w862, y=w857) -> (x+y=w867:dbl[])
          }
        }
        n263 = call-poly <vilib>:"Read Delimited Spreadsheet.vi"("file path (dialog if empty)"=path "D:/INTT/V1/Assembly Data/Tool Offsets/Bellows Tool Offset.txt", "number of rows (all:-1)"=-1) -> ("first row"=w757:dbl[])  [unwired: 8 in, 5 out]
        n264 = Index Array(array=w757, index #1=0 ("index"), index #2=1 ("index"), index #3=2 ("index")) -> (element #1=w753:dbl, element #2=w752:dbl, element #3=w751:dbl)
        n265 = for {
          N: 1 -> [_]
          tunnel: w760 -> [w766]
          tunnel: [w788] -> w750
          tunnel: w749 -> [w797] mode=indexing
          tunnel: [w775] -> w743
          tunnel: w744 -> [w765]
          tunnel: w753 -> [w790]
          tunnel: w752 -> [w789]
          tunnel: w751 -> [w787]
          tunnel: w745 -> [w781]
          tunnel: w742 -> [w768]
          tunnel: w739 -> [w767]
          tunnel: w737 -> [w763]
          w777 = 0 ("Write")
          w780 = TRUE ("Write Value")
          # "putback pickup tool"
          # "pickup tool"
          # "pickup tool height offset"
          # "Pick up PICKUP TOOL"
          # "Pick up CHIPs/Sensor and place on HDI"
          n266 = Build Array(w790, w789, w787, 0.0 ("element")) -> (w786:dbl[])
          n267 = Add(x=w797, y=w786) -> (x+y=w761:dbl[])
          n268 = call "XYZTheta-2Zspeed Go.vi"("XYZTheta In"=w761, "Motion in"=w766) -> ("error out"=w764:errorcluster, "Motion out"=w762:refnum<class "Motion.lvclass">)  [unwired: 7 in, 1 out]
          n269 = call "WriteReadWait.vi"("Read Value"=w780, "Write Value"=w780, "error in (no error)"=w764, "Read"=w777, "Write"=w777, "I-O in"=w765) -> ("error out"=w779:errorcluster, "I-O out"=w778:refnum<class "NI-DAQ.lvclass">)  [unwired: 4 in]
          n270 = Replace Array Subset(array=w786, new element=-16.0 ("t"), index=2) -> (w784:dbl[])
          n271 = for {
            N: w781 -> [_]
            tunnel: w762 -> [w809]
            tunnel: w784 -> [w808]
            tunnel: w779 -> [w807]
            tunnel: [w806] -> w791
            tunnel: w778 -> [w805]
            tunnel: [w804] -> w776
            tunnel: [w803] -> w783
            tunnel: w768 -> [w800]
            tunnel: w767 -> [w799]
            tunnel: w763 -> [w798] mode=indexing
            n272 = flat-sequence {
              tunnel: [w829] -> w810
              tunnel: w809 -> [w828]
              tunnel: w808 -> [w827]
              tunnel: w807 -> [w825]
              tunnel: w805 -> [w817]
              tunnel: [w824] -> w802
              tunnel: [w821] -> w801
              tunnel: w800 -> [w814]
              tunnel: w799 -> [w820]
              tunnel: w810 -> [w836]
              tunnel: [w844] -> w806
              tunnel: [w843] -> _
              tunnel: w808 -> [w838]
              tunnel: [w839] -> w804
              tunnel: [w834] -> w803
              tunnel: w802 -> [w841]
              tunnel: w801 -> [w835]
              tunnel: w798 -> [w837]
              frame #0 {
                w815 = FALSE ("Write Value")
                w822 = TRUE ("Write Value")
                w823 = 1 ("Write")
                # "pickup module"
                # "release module"
                # "pickup sample from tray"
                n273 = Add(x=w820, y=w827) -> (x+y=w826:dbl[])
                n274 = call "XYZTheta-2Zspeed Go.vi"("error in (no error)"=w825, "XYZTheta In"=w826, "Motion in"=w828) -> ("error out"=w818:errorcluster, "Motion out"=w829:refnum<class "Motion.lvclass">)  [unwired: 6 in, 1 out]
                n275 = call "Time Delay"("error in (no error)"=w818) -> ("error out"=w811:errorcluster)  [unwired: 10 in]
                n276 = call "0"("error in (no error)"=w811) -> ("error out"=w812:errorcluster)  [unwired: 9 in, 1 out]
                n277 = call "WriteReadWait.vi"("Read Value"=w815, "Write Value"=w815, "error in (no error)"=w812, "Read"=w814, "Write"=w814, "I-O in"=w817) -> ("error out"=w813:errorcluster, "I-O out"=w816:refnum<class "NI-DAQ.lvclass">)  [unwired: 4 in]
                n278 = call "Time Delay3"("error in (no error)"=w813) -> ("error out"=w819:errorcluster)  [unwired: 10 in]
                n279 = call "WriteReadWait.vi"("Read Value"=w822, "Write Value"=w822, "error in (no error)"=w819, "Read"=w823, "Write"=w823, "I-O in"=w816) -> ("error out"=w821:errorcluster, "I-O out"=w824:refnum<class "NI-DAQ.lvclass">)  [unwired: 4 in]
              }
              frame #1 {
                w840 = 1 ("Write")
                w842 = FALSE ("Write Value")
                # "lift for chip/sensor thickness"
                # "place sample on HDI"
                n280 = Add(x=w837, y=w838) -> (x+y=w833:dbl[])
                n281 = call "XYZTheta-2Zspeed Go.vi"("error in (no error)"=w835, "XYZTheta In"=w833, "Motion in"=w836) -> ("error out"=w832:errorcluster, "XYZTheta Out"=w843:dbl[], "Motion out"=w844:refnum<class "Motion.lvclass">)  [unwired: 6 in]
                n282 = call "1"("error in (no error)"=w832) -> ("error out"=w831:errorcluster)  [unwired: 9 in, 1 out]
                n283 = call "Time Delay6"("error in (no error)"=w831) -> ("error out"=w830:errorcluster)  [unwired: 10 in]
                n284 = call "WriteReadWait.vi"("Read Value"=w842, "Write Value"=w842, "error in (no error)"=w830, "Read"=w840, "Write"=w840, "I-O in"=w841) -> ("error out"=w834:errorcluster, "I-O out"=w839:refnum<class "NI-DAQ.lvclass">)  [unwired: 4 in]
              }
            }
          }
          n285 = call "XYZTheta-2Zspeed Go.vi"("error in (no error)"=w783, "XYZTheta In"=w761, "Motion in"=w791) -> ("error out"=w771:errorcluster, "Motion out"=w795:refnum<class "Motion.lvclass">)  [unwired: 6 in, 1 out]
          n286 = call "Time Delay9"("error in (no error)"=w771) -> ("error out"=w773:errorcluster)  [unwired: 10 in]
          n287 = call-dynamic "Digital Write 1 Channel.vi"("DAQ Module"=0, "error constant"=w773, "Value"=FALSE, "Channel"=0, "NI-DAQ.lvclass"=w776) -> ("error IO"=w772:errorcluster, "NI-DAQ.lvclass 2"=w775:refnum<class "NI-DAQ.lvclass">)  [unwired: 5 in]
          n288 = call "Time Delay10"("error in (no error)"=w772) -> ("error out"=w792:errorcluster)  [unwired: 10 in]
          n289 = call-dynamic "Z Go.vi"("error in (no error)"=w792, "Speed"=10.0, "Position"=0.0 ("new element/subarray"), "Motion in"=w795) -> ("Motion out"=w788:refnum<class "Motion.lvclass">)  [unwired: 6 in, 1 out]
        }
      }
      event "GOTO": Value Change {
        (unwired) "GOING to a position" ("String")
        n290 = event-data() -> ()  [unwired: 1 in, 6 out]
        n291 = call "XYZTheta Go.vi"("XYZTheta In"="Parking position", "Motion in"=w874) -> ("Motion out"=w872:refnum<class "Motion.lvclass">)  [unwired: 7 in, 2 out]
      }
      event "READ Position": Value Change {
        n292 = event-data() -> ()  [unwired: 1 in, 6 out]
        n293 = call-dynamic "Get Current Position.vi"("Motion in"=w892) -> ("XYZTheta Out"=→"Gantry current position":dbl[], "Motion out"=w891:refnum<class "Motion.lvclass">)  [unwired: 8 in, 1 out]
      }
      event "HDI vacuum": Value Change {
        n294 = event-data() -> ()  [unwired: 1 in, 6 out]
        n295 = call "WriteReadWait.vi"("Read Value"="vacuum", "Write Value"="vacuum", "Read"=w903, "Write"=w903, "I-O in"=w906) -> ("error out"=w904:errorcluster, "I-O out"=w893:refnum<class "NI-DAQ.lvclass">)  [unwired: 5 in]
        n296 = call "Time Delay2"("error in (no error)"=w904) -> ()  [unwired: 10 in, 1 out]
      }
      event Timeout {
        n297 = event-data() -> ()  [unwired: 1 in, 3 out]
        n298 = call-dynamic "Digital Read 1 Channel.vi"("Read"=w917, "NI-DAQ in"=w918) -> ("Value"=→"Status":bool, "NI-DAQ out"=w916:refnum<class "NI-DAQ.lvclass">)  [unwired: 7 in, 1 out]
      }
    }
    "Measured HDI size" <- w19
    "module position on stave" <- w20
    "Stave mark" <- w18
    "measured HDI top-left position" <- w15
    n299 = feedback-in #1(w19) -> ()
    n300 = feedback-in #2(w18) -> ()
    n301 = feedback-in #3(w15) -> ()
    n302 = feedback-in #4(w31) -> ()
    n303 = feedback-in #5(w28) -> ()
    n304 = feedback-in #6(w36) -> ()
    n305 = feedback-in #7(w20) -> ()
    n306 = feedback-in #8(w37) -> ()
    "# of tasks excuted" <- w33
  }
  n307 = call-dynamic "Disconnect.vi"("Controller in"=w4) -> ()  [unwired: 9 in, 1 out]
  n308 = call-dynamic "Disconnect.vi"("I-O in"=w1) -> ()  [unwired: 9 in, 1 out]
